vi "СПШ.vi"() -> ()   [LabVIEW 2010]
uses:
  <vilib>/Instr/_visa.llb/VISA Configure Serial Port (Instr).vi
panel:
  out "Serial Settings:Number of Bytes at Serial Port":u32
  out "x/y 2":dbl
  in  "Данные_16":i16
  in  "Данные_32":i32 format="%0.0f"
  in  "Банк":u16 format="%04x"
  out "x/y":dbl format="%#.1g"
  out "second subarray":u8[](array[numeric])
  out "Запрос":u8[](array[numeric])=[1, 5, 0, 30, 0, 0, 0, 0, 3] format="%02x"
  out "К-во байт":u16
  out "Адрес":u16=66 format="%04x"
  out "Тип":u8 format="%02x"
  in  "Тип запроса":T1(ring)
  in  "Форм.запроса":bool
  out "Смещение":i32[](array[numeric])
  out "Сорт парам":T2(array[cluster])=[{"Имя"="cp1", "Группа"="cp", "Наименование"="Пропорциональный коэффициент контура тока", "Ед. изм"=0, "Список"="", "Адрес"=0, "Описание"="Параметр настройки ПИ-регулятора контура тока", "Мин"=0, "Макс"=100, "Сервис"=TRUE, "Только чтение"=FALSE, "Разработка"=FALSE, "К-во бит"=32, "Шаг"=12, "Обработка"=FALSE, "Макрос"=""}, {"Имя"="cp2", "Группа"="cp", "Наименование"="Интегральный коэффициент контура тока", "Ед. изм"=0, "Список"="", "Адрес"=2, "Описание"="Параметр настройки ПИ-регулятора контура тока", "Мин"=0, "Макс"=200, "Сервис"=TRUE, "Только чтение"=FALSE, "Разработка"=FALSE, "К-во бит"=32, "Шаг"=12, "Обработка"=FALSE, "Макрос"=""}, {"Имя"="cp3", "Группа"="cp", "Наименование"="Максимальный ток", "Ед. изм"=1, "Список"="", "Адрес"=4, "Описание"="Определять предельную величину тока допустимую для двигателя.", "Мин"=0, "Макс"=1500, "Сервис"=FALSE, "Только чтение"=FALSE, "Разработка"=FALSE, "К-во бит"=16, "Шаг"=0, "Обработка"=TRUE, "Макрос"="macros cp3\n  ON_READ\n  READ cp3\n  cp3=cp3*5/2047\n  RETURN cp3\n  ON_WRITE\n  cp3=val*2047/5\n  WRITE cp3\nend"}, {"Имя"="cp4", "Группа"="cp", "Наименование"="Максимальная скваженность ШИМ", "Ед. изм"=1, "Список"="", "Адрес"=5, "Описание"="3070 дискрет соответствует 100% заполнения", "Мин"=0, "Макс"=6150, "Сервис"=FALSE, "Только чтение"=FALSE, "Разработка"=FALSE, "К-во бит"=16, "Шаг"=0, "Обработка"=TRUE, "Макрос"="macros cp4\n  ON_READ\n  READ cp4\n  cp4=cp4*5/2500\n  RETURN cp4\n  ON_WRITE\n  cp4=val*2500/5\n  WRITE cp4\nend"}, {"Имя"="vp1", "Группа"="vp", "Наименование"="Пропорциональный коэффициент контура скорости", "Ед. изм"=0, "Список"="", "Адрес"=6, "Описание"="Параметр настройки ПИ-регулятора контура скорости", "Мин"=0, "Макс"=60000, "Сервис"=TRUE, "Только чтение"=FALSE, "Разработка"=FALSE, "К-во бит"=32, "Шаг"=12, "Обработка"=FALSE, "Макрос"=""}, {"Имя"="vp2", "Группа"="vp", "Наименование"="Интегральный коэффициент контура скорости", "Ед. изм"=0, "Список"="", "Адрес"=7, "Описание"="Параметр настройки ПИ-регулятора контура скорости", "Мин"=0, "Макс"=60000, "Сервис"=TRUE, "Только чтение"=FALSE, "Разработка"=FALSE, "К-во бит"=32, "Шаг"=12, "Обработка"=FALSE, "Макрос"=""}, {"Имя"="vp16", "Группа"="vp", "Наименование"="Дифференциальный коэффициент контура скорости", "Ед. изм"=0, "Список"="", "Адрес"=80, "Описание"="Параметр настройки ПИ-регулятора контура скорости", "Мин"=0, "Макс"=60000, "Сервис"=TRUE, "Только чтение"=FALSE, "Разработка"=FALSE, "К-во бит"=32, "Шаг"=12, "Обработка"=FALSE, "Макрос"=""}, {"Имя"="vp3", "Группа"="vp", "Наименование"="Коэффициент обратной связи по скорости", "Ед. изм"=0, "Список"="", "Адрес"=8, "Описание"="Определяет масштаб датчика скорости", "Мин"=-1, "Макс"=1, "Сервис"=TRUE, "Только чтение"=FALSE, "Разработка"=FALSE, "К-во бит"=32, "Шаг"=12, "Обработка"=FALSE, "Макрос"=""}, {"Имя"="vp4", "Группа"="vp", "Наименование"="Частота дискретизации контура скорости", "Ед. изм"=0, "Список"="100:100\n 200:200\n 500:500\n 1000:1000\n 2000:2000\n 3000:3000\n 4000:4000\n 5000:5000\n\r\n", "Адрес"=9, "Описание"="Определяет частоту обсчета контура скорости", "Мин"=100, "Макс"=5000, "Сервис"=FALSE, "Только чтение"=FALSE, "Разработка"=FALSE, "К-во бит"=16, "Шаг"=0, "Обработка"=FALSE, "Макрос"=""}, {"Имя"="vp5", "Группа"="vp", "Наименование"="Ускорение", "Ед. изм"=2, "Список"="", "Адрес"=10, "Описание"="Определяет динамику контура скорости", "Мин"=1, "Макс"=2000000, "Сервис"=TRUE, "Только чтение"=FALSE, "Разработка"=FALSE, "К-во бит"=32, "Шаг"=10, "Обработка"=FALSE, "Макрос"=""}, {"Имя"="pp1", "Группа"="pp", "Наименование"="Пропорциональный коэффициент контура положения", "Ед. изм"=0, "Список"="", "Адрес"=11, "Описание"="Параметр настройки ПИ-регулятора контура позиционирования", "Мин"=0, "Макс"=10000, "Сервис"=TRUE, "Только чтение"=FALSE, "Разработка"=FALSE, "К-во бит"=32, "Шаг"=4, "Обработка"=FALSE, "Макрос"=""}, {"Имя"="pp2", "Группа"="pp", "Наименование"="Интегральный коэффициент контура положения", "Ед. изм"=0, "Список"="", "Адрес"=12, "Описание"="Параметр настройки ПИ-регулятора контура позиционирования", "Мин"=0, "Макс"=30000, "Сервис"=TRUE, "Только чтение"=FALSE, "Разработка"=FALSE, "К-во бит"=32, "Шаг"=4, "Обработка"=FALSE, "Макрос"=""}, {"Имя"="pp3", "Группа"="pp", "Наименование"="Частота дискретизации контура положения", "Ед. изм"=0, "Список"="25:25\n50:50\n100:100\n200:200\n500:500\n1000:1000\n2000:2000\n3000:3000\n4000:4000\n5000:5000\n\r\n", "Адрес"=13, "Описание"="Определяет частоту обсчета контура позиции.", "Мин"=25, "Макс"=5000, "Сервис"=FALSE, "Только чтение"=FALSE, "Разработка"=FALSE, "К-во бит"=16, "Шаг"=0, "Обработка"=FALSE, "Макрос"=""}, {"Имя"="vp6", "Группа"="vp", "Наименование"="Максимальное время выхода на номинальный режим", "Ед. изм"=3, "Список"="0:Не ограничено\n1:1\n2:2\n3:3\n4:4\n5:5\n6:6\n7:7\n8:8\n9:9\n10:10\n11:11\n12:12\n13:13\n14:14\n15:15\n16:16\n17:17\n18:18\n19:19\n20:20\n21:21\n22:22\n23:23\n24:24\n25:25\n26:26\n27:27\n28:28\n29:29\n30:30\r\n", "Адрес"=14, "Описание"="Время, по истечению которого привод переходит в состояние останова, если не достигнута заданная скорость", "Мин"=0, "Макс"=30, "Сервис"=FALSE, "Только чтение"=FALSE, "Разработка"=FALSE, "К-во бит"=16, "Шаг"=1, "Обработка"=TRUE, "Макрос"="macros vp6\n  ON_READ\n  READ vp6\n  if vp4=0\n  READ vp4\n  fi\n  vp6=vp6/vp4\n  RETURN vp6\n  ON_WRITE\n  if vp4=0\n  READ vp4\n  fi\n  vp6=val*vp4\n  WRITE vp6\n  ON_ERROR\n  vp6=100000000000000\n  RETURN vp6\nend"}, {"Имя"="cp5", "Группа"="cp", "Наименование"="Состояние контура тока", "Ед. изм"=0, "Список"="0:Разомкнут\n2:Замкнут\n4:Прямое управление токами в обмотках\n5:Адаптивное упрваление\n6:Прямое раздельное управление токами в обмотках\n\r\n", "Адрес"=16, "Описание"="Обеспечивает замкнутое или разомкнутое регулирование контура тока. В стандартном режиме использования контур должен быть замкнут.", "Мин"=0, "Макс"=6, "Сервис"=FALSE, "Только чтение"=FALSE, "Разработка"=FALSE, "К-во бит"=16, "Шаг"=0, "Обработка"=FALSE, "Макрос"=""}, {"Имя"="vp7", "Группа"="vp", "Наименование"="Состояние контура скорости", "Ед. изм"=0, "Список"="0:Разомкнут\n2:Замкнут\n\r\n", "Адрес"=17, "Описание"="Обеспечивает замкнутое или разомкнутое регулирование контура скорости. Контур должен быть замкнут в режиме управления скоростью привода и в режиме управления позицией.", "Мин"=0, "Макс"=2, "Сервис"=FALSE, "Только чтение"=FALSE, "Разработка"=FALSE, "К-во бит"=16, "Шаг"=0, "Обработка"=FALSE, "Макрос"=""}, {"Имя"="pp5", "Группа"="pp", "Наименование"="Состояние контура положения", "Ед. изм"=0, "Список"="0:Разомкнут\n2:Замкнут\n\r\n", "Адрес"=18, "Описание"="Обеспечивает замкнутое или разомкнутое регулирование контура позиции", "Мин"=0, "Макс"=2, "Сервис"=FALSE, "Только чтение"=FALSE, "Разработка"=FALSE, "К-во бит"=16, "Шаг"=0, "Обработка"=FALSE, "Макрос"=""}, {"Имя"="vp8", "Группа"="vp", "Наименование"="Максимальная скорость вращения", "Ед. изм"=4, "Список"="", "Адрес"=20, "Описание"="Ограничение максимальной скорости вращения привода.", "Мин"=0, "Макс"=8000, "Сервис"=TRUE, "Только чтение"=FALSE, "Разработка"=FALSE, "К-во бит"=32, "Шаг"=12, "Обработка"=FALSE, "Макрос"=""}, {"Имя"="vp9", "Группа"="vp", "Наименование"="Динамический режим", "Ед. изм"=0, "Список"="0:Режим плавного разгона/торможения\n2:Режим с максимальной динамикой\n3:Режим G декодирования\n4:S кривая\n\r\n", "Адрес"=15, "Описание"="Включает или отключает внутренний интерполятор. В режиме управления приводов от внешнего контроллера, например, от ЧПУ, привод должен находиться в режиме с максимальной динамикой. Режим G декодирования позволяет реализовать контурное управление непосредственно группой приводов без использования внешнего контроллера.", "Мин"=0, "Макс"=4, "Сервис"=FALSE, "Только чтение"=FALSE, "Разработка"=FALSE, "К-во бит"=16, "Шаг"=0, "Обработка"=FALSE, "Макрос"=""}, {"Имя"="ss1", "Группа"="ss", "Наименование"="Тестовый параметр", "Ед. изм"=0, "Список"="", "Адрес"=19, "Описание"="", "Мин"=-65535, "Макс"=65535, "Сервис"=FALSE, "Только чтение"=FALSE, "Разработка"=TRUE, "К-во бит"=16, "Шаг"=0, "Обработка"=FALSE, "Макрос"=""}, {"Имя"="ct1", "Группа"="ct", "Наименование"="Задание тока", "Ед. изм"=5, "Список"="", "Адрес"=512, "Описание"="Сигнал управления при разомкнутом контуре скорости и положения", "Мин"=-3500, "Макс"=3500, "Сервис"=FALSE, "Только чтение"=FALSE, "Разработка"=FALSE, "К-во бит"=16, "Шаг"=0, "Обработка"=TRUE, "Макрос"="macros ct1\n  ON_READ\n  READ ct1\n  ct1=ct1*5/2500\n  RETURN ct1\n  ON_WRITE\n  ct1=val*2500/5\n  WRITE ct1\nend"}, {"Имя"="ct2", "Группа"="ct", "Наименование"="Задание скорости", "Ед. изм"=4, "Список"="", "Адрес"=514, "Описание"="Сигнал управления при разомкнутом контуре положения", "Мин"=-12000, "Макс"=12000, "Сервис"=TRUE, "Только чтение"=FALSE, "Разработка"=FALSE, "К-во бит"=32, "Шаг"=12, "Обработка"=FALSE, "Макрос"=""}, {"Имя"="ct3", "Группа"="ct", "Наименование"="Задание положения", "Ед. изм"=6, "Список"="", "Адрес"=516, "Описание"="Сигнал управления при замкнутом контуре положения", "Мин"=-2147483647, "Макс"=2147483647, "Сервис"=FALSE, "Только чтение"=FALSE, "Разработка"=FALSE, "К-во бит"=32, "Шаг"=0, "Обработка"=FALSE, "Макрос"=""}, {"Имя"="dd1", "Группа"="dd", "Наименование"="Ток в обмотке 1", "Ед. изм"=5, "Список"="", "Адрес"=1024, "Описание"="Показывает ток, протекающий в обмотке двигателя", "Мин"=-5, "Макс"=5, "Сервис"=FALSE, "Только чтение"=TRUE, "Разработка"=FALSE, "К-во бит"=16, "Шаг"=0, "Обработка"=TRUE, "Макрос"="macros dd1\n  ON_READ\n  READ dd1\n  dd1=dd1*5/2047\n  RETURN dd1\n  ON_WRITE\n  dd1=val*2047/5\n  WRITE dd1\nend"}, {"Имя"="dd6", "Группа"="dd", "Наименование"="Заданный ток в обмотке 1", "Ед. изм"=5, "Список"="", "Адрес"=1034, "Описание"="", "Мин"=-2047, "Макс"=2047, "Сервис"=FALSE, "Только чтение"=FALSE, "Разработка"=FALSE, "К-во бит"=16, "Шаг"=0, "Обработка"=TRUE, "Макрос"="macros dd6\n  ON_READ\n  READ dd6\n  dd6=dd6*5/2047\n  RETURN dd6\n  ON_WRITE\n  dd6=val*2047/5\n  WRITE dd6\nend"}, {"Имя"="dd3", "Группа"="dd", "Наименование"="Ток в обмотке 2", "Ед. изм"=5, "Список"="", "Адрес"=1029, "Описание"="Индицирует ток, протекающий в обмотке двигателя", "Мин"=-5, "Макс"=5, "Сервис"=FALSE, "Только чтение"=TRUE, "Разработка"=FALSE, "К-во бит"=16, "Шаг"=0, "Обработка"=TRUE, "Макрос"="macros dd3\n  ON_READ\n  READ dd3\n  dd3=dd3*5/2047\n  RETURN dd3\n  ON_WRITE\n  dd3=val*2047/5\n  WRITE dd3\nend"}, {"Имя"="dd9", "Группа"="dd", "Наименование"="Заданный ток в обмотке 2", "Ед. изм"=5, "Список"="", "Адрес"=1037, "Описание"="", "Мин"=-2047, "Макс"=2047, "Сервис"=FALSE, "Только чтение"=FALSE, "Разработка"=FALSE, "К-во бит"=16, "Шаг"=0, "Обработка"=TRUE, "Макрос"="macros dd9\n  ON_READ\n  READ dd9\n  dd9=dd9*5/2047\n  RETURN dd9\n  ON_WRITE\n  dd9=val*2047/5\n  WRITE dd9\nend"}, {"Имя"="dd2", "Группа"="dd", "Наименование"="Заданный ток в роторной системе координат", "Ед. изм"=5, "Список"="", "Адрес"=1026, "Описание"="Индицирует ток, который задан контуром скорости", "Мин"=-5, "Макс"=5, "Сервис"=FALSE, "Только чтение"=TRUE, "Разработка"=FALSE, "К-во бит"=16, "Шаг"=0, "Обработка"=TRUE, "Макрос"="macros dd2\n  ON_READ\n  READ dd2\n  dd2=dd2*5/2047\n  RETURN dd2\n  ON_WRITE\n  dd2=val*2047/5\n  WRITE dd2\nend"}, {"Имя"="dd4", "Группа"="dd", "Наименование"="Текущая скорость вращения", "Ед. изм"=4, "Список"="", "Адрес"=1032, "Описание"="", "Мин"=-5000, "Макс"=5000, "Сервис"=FALSE, "Только чтение"=TRUE, "Разработка"=FALSE, "К-во бит"=8, "Шаг"=12, "Обработка"=FALSE, "Макрос"=""}, {"Имя"="dd5", "Группа"="dd", "Наименование"="Заданная скорость вращения", "Ед. изм"=4, "Список"="", "Адрес"=1033, "Описание"="", "Мин"=-5000, "Макс"=5000, "Сервис"=FALSE, "Только чтение"=TRUE, "Разработка"=FALSE, "К-во бит"=16, "Шаг"=12, "Обработка"=FALSE, "Макрос"=""}, {"Имя"="dd21", "Группа"="dd", "Наименование"="Ошибка контура скорости", "Ед. изм"=4, "Список"="", "Адрес"=1049, "Описание"="", "Мин"=-65535, "Макс"=65535, "Сервис"=FALSE, "Только чтение"=TRUE, "Разработка"=FALSE, "К-во бит"=16, "Шаг"=1, "Обработка"=FALSE, "Макрос"=""}, {"Имя"="dd7", "Группа"="dd", "Наименование"="Заданная позиция", "Ед. изм"=6, "Список"="", "Адрес"=1035, "Описание"="", "Мин"=-2147483647, "Макс"=2147483647, "Сервис"=FALSE, "Только чтение"=TRUE, "Разработка"=FALSE, "К-во бит"=32, "Шаг"=0, "Обработка"=FALSE, "Макрос"=""}, {"Имя"="dd8", "Группа"="dd", "Наименование"="Текущая позиция", "Ед. изм"=6, "Список"="", "Адрес"=1036, "Описание"="", "Мин"=-2147483647, "Макс"=2147483647, "Сервис"=FALSE, "Только чтение"=TRUE, "Разработка"=FALSE, "К-во бит"=32, "Шаг"=0, "Обработка"=FALSE, "Макрос"=""}, {"Имя"="dd20", "Группа"="dd", "Наименование"="Ошибка контура позиции", "Ед. изм"=6, "Список"="", "Адрес"=1048, "Описание"="", "Мин"=-2147483647, "Макс"=2147483647, "Сервис"=TRUE, "Только чтение"=TRUE, "Разработка"=FALSE, "К-во бит"=32, "Шаг"=10, "Обработка"=FALSE, "Макрос"=""}, {"Имя"="dd10", "Группа"="dd", "Наименование"="Температура внутри корпуса", "Ед. изм"=7, "Список"="", "Адрес"=1038, "Описание"="", "Мин"=-40, "Макс"=120, "Сервис"=FALSE, "Только чтение"=TRUE, "Разработка"=FALSE, "К-во бит"=16, "Шаг"=0, "Обработка"=TRUE, "Макрос"="macros dd10\n  ON_READ\n  READ dd10\n  dd10=dd10/128\n  RETURN dd10\n  ON_WRITE\n  dd10=val\n  WRITE dd10\nend"}, {"Имя"="dd19", "Группа"="dd", "Наименование"="Текущее цифровое напряжение", "Ед. изм"=8, "Список"="", "Адрес"=1047, "Описание"="", "Мин"=0, "Макс"=23, "Сервис"=FALSE, "Только чтение"=TRUE, "Разработка"=FALSE, "К-во бит"=16, "Шаг"=0, "Обработка"=TRUE, "Макрос"="macros dd19\n  ON_READ\n  READ dd19\n  dd19=dd19/178\n  RETURN dd19\n  ON_WRITE\n  dd19=val\n  WRITE dd19\nend"}, {"Имя"="dd12", "Группа"="dd", "Наименование"="Текущее напряжение питания", "Ед. изм"=8, "Список"="", "Адрес"=1040, "Описание"="", "Мин"=0, "Макс"=120, "Сервис"=FALSE, "Только чтение"=TRUE, "Разработка"=FALSE, "К-во бит"=16, "Шаг"=0, "Обработка"=TRUE, "Макрос"="macros dd12\n  ON_READ\n  READ dd12\n  dd12=dd12/21\n  RETURN dd12\n  ON_WRITE\n  dd12=val\n  WRITE dd12\nend"}, {"Имя"="dd11", "Группа"="dd", "Наименование"="Статус контроллера", "Ед. изм"=0, "Список"="0:Исправен\n1:Останов по команде\n2:Останов - высокое противодействующее усилие\n3:Останов - короткое замыкание\n4:Выход из температурного диапазона\n5:Повышенное силовое напряжение\n6:Низкое силовое напряжение\n7:Повышенное цифровое напряжение\n8:Низкое цифровое напряжение\n9:Cиловое напряжение превышает напряжение, установл. пользователем\n10:Останов - превышение допустимой перегрузки\n11:Останов - сработала защита IGBT модуля\n12:Останов - Ошибка поиска фазы по UVW трекам\n13:Останов - ошибка в настройках энкодера\n14: Останов - сбой в работе энкодера\n15: Останов - Ошибка фазировки двигателя\n\r\n", "Адрес"=1039, "Описание"="Привод в состоянии отработать задание только, если его статус \"Исправен\".", "Мин"=0, "Макс"=15, "Сервис"=FALSE, "Только чтение"=FALSE, "Разработка"=FALSE, "К-во бит"=16, "Шаг"=0, "Обработка"=FALSE, "Макрос"=""}, {"Имя"="st1", "Группа"="st", "Наименование"="Разрешение", "Ед. изм"=6, "Список"="", "Адрес"=21, "Описание"="Разрешение датчика положения/скорости", "Мин"=0, "Макс"=2147483647, "Сервис"=FALSE, "Только чтение"=FALSE, "Разработка"=FALSE, "К-во бит"=32, "Шаг"=0, "Обработка"=FALSE, "Макрос"=""}, {"Имя"="tp1", "Группа"="tp", "Наименование"="Режим осциллографа", "Ед. изм"=0, "Список"="0:Непрерывный режим\n1:Ступенька\n2:Синус\n3:Приращение скорости\n4:Синусоидальное изменение скорости\n5:Треугольное изменение позиции\n6:Измерение без задания\n7:Измерение без задания до принудительного останова\n8:Приращение момента\n\r\n", "Адрес"=1280, "Описание"="Режим сканирования динамических параметров (отображение выбранных параметров в процессе работы привода).", "Мин"=0, "Макс"=8, "Сервис"=FALSE, "Только чтение"=FALSE, "Разработка"=FALSE, "К-во бит"=16, "Шаг"=0, "Обработка"=FALSE, "Макрос"=""}, {"Имя"="tp3", "Группа"="tp", "Наименование"="Амплитуда задания положения", "Ед. изм"=0, "Список"="", "Адрес"=1284, "Описание"="Определяет величину приращения позиции в режиме осциллографа 1.", "Мин"=-2147483647, "Макс"=2147483647, "Сервис"=FALSE, "Только чтение"=FALSE, "Разработка"=FALSE, "К-во бит"=32, "Шаг"=0, "Обработка"=FALSE, "Макрос"=""}, {"Имя"="ip0", "Группа"="ip", "Наименование"="Источник опорного сигнала", "Ед. изм"=0, "Список"="0:Интерфейс USB\n2:Интерфейс StepDir\n4:Аналоговый интерфейс\n5:Интерфейс CAN\n6:Квадратурный интерфейс\r\n", "Адрес"=23, "Описание"="Определяет интерфейс, по которому осуществляется ввод задания для привода.", "Мин"=0, "Макс"=6, "Сервис"=FALSE, "Только чтение"=FALSE, "Разработка"=FALSE, "К-во бит"=16, "Шаг"=0, "Обработка"=FALSE, "Макрос"=""}, {"Имя"="st2", "Группа"="st", "Наименование"="Версия ПО драйвера", "Ед. изм"=0, "Список"="", "Адрес"=22, "Описание"="Текущая версия программного обеспечения привода.", "Мин"=0, "Макс"=2147483647, "Сервис"=TRUE, "Только чтение"=FALSE, "Разработка"=FALSE, "К-во бит"=32, "Шаг"=12, "Обработка"=FALSE, "Макрос"=""}, {"Имя"="ip1", "Группа"="ip", "Наименование"="Коэффициент веса одной дискреты", "Ед. изм"=0, "Список"="", "Адрес"=24, "Описание"="Определяет количество импульсов датчика, на которые необходимо повернуть вал двигателя, при получении одной дискреты по интерфейсу Step/Dir, т.е. масштаб одного импульса", "Мин"=-4000, "Макс"=4000, "Сервис"=TRUE, "Только чтение"=FALSE, "Разработка"=FALSE, "К-во бит"=32, "Шаг"=10, "Обработка"=FALSE, "Макрос"=""}, {"Имя"="tp2", "Группа"="tp", "Наименование"="Период опроса параметров", "Ед. изм"=9, "Список"="", "Адрес"=1282, "Описание"="Определяет интервал времени между запоминанием данных в массив в режимах 1-7.", "Мин"=25, "Макс"=25000, "Сервис"=FALSE, "Только чтение"=FALSE, "Разработка"=FALSE, "К-во бит"=16, "Шаг"=25, "Обработка"=FALSE, "Макрос"=""}, {"Имя"="tp5", "Группа"="tp", "Наименование"="Период задающего воздействия", "Ед. изм"=9, "Список"="", "Адрес"=1285, "Описание"="Данный параметр определяет задержку введения задающего воздействия от начала сбора информации в режиме осциллографа 1 и 3.", "Мин"=25, "Макс"=800000, "Сервис"=FALSE, "Только чтение"=FALSE, "Разработка"=FALSE, "К-во бит"=16, "Шаг"=25, "Обработка"=TRUE, "Макрос"="macros tp5\n  ON_READ\n  READ tp5\n  tp5=tp5*25\n  RETURN tp5\n  ON_WRITE\n  tp5=val/25\n  WRITE tp5\n  ON_ERROR\n  err=100000000000\n  RETURN err\nend"}, {"Имя"="tp6", "Группа"="tp", "Наименование"="Амплитуда задания скорости", "Ед. изм"=4, "Список"="", "Адрес"=1286, "Описание"="Определяет величину приращения скорости в режиме осциллографа 3.", "Мин"=-14000, "Макс"=14000, "Сервис"=FALSE, "Только чтение"=FALSE, "Разработка"=FALSE, "К-во бит"=16, "Шаг"=0, "Обработка"=FALSE, "Макрос"=""}, {"Имя"="ip2", "Группа"="ip", "Наименование"="Текущий банк программы интерпретатора", "Ед. изм"=10, "Список"="0:0\n1:1\n2:2\n3:3\n4:4\n5:5\n6:6\n7:7\n255:Программа не выбрана\n\r\n", "Адрес"=26, "Описание"="Банк, из которой загружена программа на выполнение.", "Мин"=0, "Макс"=255, "Сервис"=FALSE, "Только чтение"=FALSE, "Разработка"=FALSE, "К-во бит"=16, "Шаг"=1, "Обработка"=FALSE, "Макрос"=""}, {"Имя"="ip3", "Группа"="ip", "Наименование"="Текущий банк чт/записи программ интерпретатора", "Ед. изм"=10, "Список"="0:0\n1:1\n2:2\n3:3\n4:4\n5:5\n6:6\n7:7\n255:Программа не выбрана\n\r\n", "Адрес"=27, "Описание"="", "Мин"=0, "Макс"=255, "Сервис"=FALSE, "Только чтение"=TRUE, "Разработка"=TRUE, "К-во бит"=16, "Шаг"=1, "Обработка"=FALSE, "Макрос"=""}, {"Имя"="ip4", "Группа"="ip", "Наименование"="Режим работы интерпретатора", "Ед. изм"=0, "Список"="0:Режим выполнения программы\n1:Режим отладки\n\r\n", "Адрес"=28, "Описание"="Режим работы интерпретатора", "Мин"=0, "Макс"=1, "Сервис"=FALSE, "Только чтение"=FALSE, "Разработка"=FALSE, "К-во бит"=16, "Шаг"=1, "Обработка"=FALSE, "Макрос"=""}, {"Имя"="st3", "Группа"="st", "Наименование"="Уникальный идентификатор устройства", "Ед. изм"=0, "Список"="", "Адрес"=30, "Описание"="", "Мин"=0, "Макс"=2147483647, "Сервис"=FALSE, "Только чтение"=FALSE, "Разработка"=FALSE, "К-во бит"=32, "Шаг"=0, "Обработка"=FALSE, "Макрос"=""}, {"Имя"="ip5", "Группа"="ip", "Наименование"="Порт ввода вывода", "Ед. изм"=0, "Список"="", "Адрес"=29, "Описание"="Старший байт содержит содержимое порта вывода, младший - состояние линий ввода.", "Мин"=0, "Макс"=65535, "Сервис"=FALSE, "Только чтение"=FALSE, "Разработка"=FALSE, "К-во бит"=16, "Шаг"=0, "Обработка"=FALSE, "Макрос"=""}, {"Имя"="ss2", "Группа"="ss", "Наименование"="Количество КЗ", "Ед. изм"=0, "Список"="", "Адрес"=31, "Описание"="Количество зафиксированных коротких замыканий", "Мин"=0, "Макс"=65535, "Сервис"=FALSE, "Только чтение"=FALSE, "Разработка"=FALSE, "К-во бит"=16, "Шаг"=0, "Обработка"=FALSE, "Макрос"=""}, {"Имя"="ss3", "Группа"="ss", "Наименование"="Количество превышений температуры", "Ед. изм"=0, "Список"="", "Адрес"=32, "Описание"="Количество зафиксированных превышений температуры", "Мин"=0, "Макс"=65535, "Сервис"=FALSE, "Только чтение"=FALSE, "Разработка"=FALSE, "К-во бит"=16, "Шаг"=0, "Обработка"=FALSE, "Макрос"=""}, {"Имя"="ss4", "Группа"="ss", "Наименование"="Количество перенапряжений", "Ед. изм"=0, "Список"="", "Адрес"=33, "Описание"="Количество зафиксированных перенапряжений", "Мин"=0, "Макс"=65535, "Сервис"=FALSE, "Только чтение"=FALSE, "Разработка"=FALSE, "К-во бит"=16, "Шаг"=0, "Обработка"=FALSE, "Макрос"=""}, {"Имя"="ss5", "Группа"="ss", "Наименование"="Количество недонапряжений", "Ед. изм"=0, "Список"="", "Адрес"=34, "Описание"="Количество зафиксированных случаев пониженного напряжений", "Мин"=0, "Макс"=65535, "Сервис"=FALSE, "Только чтение"=FALSE, "Разработка"=FALSE, "К-во бит"=16, "Шаг"=0, "Обработка"=FALSE, "Макрос"=""}, {"Имя"="ss6", "Группа"="ss", "Наименование"="Количество перегрузок", "Ед. изм"=0, "Список"="", "Адрес"=35, "Описание"="", "Мин"=0, "Макс"=65535, "Сервис"=FALSE, "Только чтение"=FALSE, "Разработка"=FALSE, "К-во бит"=16, "Шаг"=0, "Обработка"=FALSE, "Макрос"=""}, {"Имя"="ss7", "Группа"="ss", "Наименование"="Количество перепрогарммирований", "Ед. изм"=0, "Список"="", "Адрес"=36, "Описание"="", "Мин"=0, "Макс"=65535, "Сервис"=FALSE, "Только чтение"=FALSE, "Разработка"=FALSE, "К-во бит"=16, "Шаг"=0, "Обработка"=FALSE, "Макрос"=""}, {"Имя"="ss8", "Группа"="ss", "Наименование"="Сообщение 0", "Ед. изм"=0, "Список"="1:Короткое замыкание\n2:Перегрев\n3:Повышенное напряжение\n4:Пониженное напряжение\n5:Перегрузка по току\n6:Произведена перезапись контроллера\n\r\n", "Адрес"=37, "Описание"="Журнал последних 8 сообщений", "Мин"=0, "Макс"=65535, "Сервис"=FALSE, "Только чтение"=FALSE, "Разработка"=FALSE, "К-во бит"=16, "Шаг"=0, "Обработка"=FALSE, "Макрос"=""}, {"Имя"="ss9", "Группа"="ss", "Наименование"="Сообщение 1", "Ед. изм"=0, "Список"="1:Короткое замыкание\n2:Перегрев\n3:Повышенное напряжение\n4:Пониженное напряжение\n5:Перегрузка по току\n6:Произведена перезапись контроллера\n\r\n", "Адрес"=38, "Описание"="Журнал последних 8 сообщений", "Мин"=0, "Макс"=65535, "Сервис"=FALSE, "Только чтение"=FALSE, "Разработка"=FALSE, "К-во бит"=16, "Шаг"=0, "Обработка"=FALSE, "Макрос"=""}, {"Имя"="ss10", "Группа"="ss", "Наименование"="Сообщение 2", "Ед. изм"=0, "Список"="1:Короткое замыкание\n2:Перегрев\n3:Повышенное напряжение\n4:Пониженное напряжение\n5:Перегрузка по току\n6:Произведена перезапись контроллера\n\r\n", "Адрес"=39, "Описание"="Журнал последних 8 сообщений", "Мин"=0, "Макс"=65535, "Сервис"=FALSE, "Только чтение"=FALSE, "Разработка"=FALSE, "К-во бит"=16, "Шаг"=0, "Обработка"=FALSE, "Макрос"=""}, {"Имя"="ss11", "Группа"="ss", "Наименование"="Сообщение 3", "Ед. изм"=0, "Список"="1:Короткое замыкание\n2:Перегрев\n3:Повышенное напряжение\n4:Пониженное напряжение\n5:Перегрузка по току\n6:Произведена перезапись контроллера\n\r\n", "Адрес"=40, "Описание"="Журнал последних 8 сообщений", "Мин"=0, "Макс"=65535, "Сервис"=FALSE, "Только чтение"=FALSE, "Разработка"=FALSE, "К-во бит"=16, "Шаг"=0, "Обработка"=FALSE, "Макрос"=""}, {"Имя"="ss12", "Группа"="ss", "Наименование"="Сообщение 4", "Ед. изм"=0, "Список"="1:Короткое замыкание\n2:Перегрев\n3:Повышенное напряжение\n4:Пониженное напряжение\n5:Перегрузка по току\n6:Произведена перезапись контроллера\n\r\n", "Адрес"=41, "Описание"="Журнал последних 8 сообщений", "Мин"=0, "Макс"=65535, "Сервис"=FALSE, "Только чтение"=FALSE, "Разработка"=FALSE, "К-во бит"=16, "Шаг"=0, "Обработка"=FALSE, "Макрос"=""}, {"Имя"="ss13", "Группа"="ss", "Наименование"="Сообщение 5", "Ед. изм"=0, "Список"="1:Короткое замыкание\n2:Перегрев\n3:Повышенное напряжение\n4:Пониженное напряжение\n5:Перегрузка по току\n6:Произведена перезапись контроллера\n\r\n", "Адрес"=42, "Описание"="Журнал последних 8 сообщений", "Мин"=0, "Макс"=65535, "Сервис"=FALSE, "Только чтение"=FALSE, "Разработка"=FALSE, "К-во бит"=16, "Шаг"=0, "Обработка"=FALSE, "Макрос"=""}, {"Имя"="ss14", "Группа"="ss", "Наименование"="Сообщение 6", "Ед. изм"=0, "Список"="1:Короткое замыкание\n2:Перегрев\n3:Повышенное напряжение\n4:Пониженное напряжение\n5:Перегрузка по току\n6:Произведена перезапись контроллера\n\r\n", "Адрес"=43, "Описание"="Журнал последних 8 сообщений", "Мин"=0, "Макс"=65535, "Сервис"=FALSE, "Только чтение"=FALSE, "Разработка"=FALSE, "К-во бит"=16, "Шаг"=0, "Обработка"=FALSE, "Макрос"=""}, {"Имя"="ss15", "Группа"="ss", "Наименование"="Сообщение 7", "Ед. изм"=0, "Список"="1:Короткое замыкание\n2:Перегрев\n3:Повышенное напряжение\n4:Пониженное напряжение\n5:Перегрузка по току\n6:Произведена перезапись контроллера\n\r\n", "Адрес"=44, "Описание"="Журнал последних 8 сообщений", "Мин"=0, "Макс"=65535, "Сервис"=FALSE, "Только чтение"=FALSE, "Разработка"=FALSE, "К-во бит"=16, "Шаг"=0, "Обработка"=FALSE, "Макрос"=""}, {"Имя"="ip6", "Группа"="ip", "Наименование"="Смещение диапазона сигнала управления", "Ед. изм"=0, "Список"="", "Адрес"=48, "Описание"="Используется для корректировки диапазона регулирования входного сигнала (аналогового или Step\\Dir). Значение 2048 соответствует нулевой скорости при подаче на вход нулевого напряжения.", "Мин"=0, "Макс"=4096, "Сервис"=FALSE, "Только чтение"=FALSE, "Разработка"=FALSE, "К-во бит"=16, "Шаг"=0, "Обработка"=FALSE, "Макрос"=""}, {"Имя"="dd13", "Группа"="dd", "Наименование"="Тестовый параметр 1", "Ед. изм"=0, "Список"="", "Адрес"=1041, "Описание"="Пока используется для индикации перехода на меандр вместо синуса. Параметр для разработчика", "Мин"=-65535, "Макс"=65535, "Сервис"=FALSE, "Только чтение"=TRUE, "Разработка"=TRUE, "К-во бит"=16, "Шаг"=0, "Обработка"=FALSE, "Макрос"=""}, {"Имя"="dd14", "Группа"="dd", "Наименование"="Тестовый параметр 2", "Ед. изм"=0, "Список"="", "Адрес"=1042, "Описание"="Пока используется для индикации сдвига фазы", "Мин"=-65535, "Макс"=65535, "Сервис"=FALSE, "Только чтение"=TRUE, "Разработка"=TRUE, "К-во бит"=16, "Шаг"=0, "Обработка"=FALSE, "Макрос"=""}, {"Имя"="vp10", "Группа"="vp", "Наименование"="Начало резонансного диапазона 1", "Ед. изм"=4, "Список"="", "Адрес"=49, "Описание"="Если начало и конец диапазона равны, то диапазон не выбран.", "Мин"=0, "Макс"=8000, "Сервис"=FALSE, "Только чтение"=FALSE, "Разработка"=FALSE, "К-во бит"=16, "Шаг"=0, "Обработка"=TRUE, "Макрос"="macros vp10\n  ON_READ\n  READ vp10\n  if st1=0\n  READ st1\n  fi\n  if vp4=0\n  READ vp4\n  fi\n  if vp3=0\n  READ vp3\n  fi\n  vp10=round(60*vp10*vp4/(st1*vp3))\n  RETURN vp10\n  ON_WRITE\n  if st1=0\n  READ st1\n  fi\n  if vp4=0\n  READ vp4\n  fi\n  if vp3=0\n  READ vp3\n  fi\n  vp10=val*st1*vp3/(60*vp4)\n  WRITE vp10\n  ON_ERROR\n  vp10=100000000000000\n  RETURN vp10\nend"}, {"Имя"="vp11", "Группа"="vp", "Наименование"="Конец резонансного диапазона 1", "Ед. изм"=4, "Список"="", "Адрес"=50, "Описание"="Если начало и конец диапазона равны, то диапазон не выбран.", "Мин"=0, "Макс"=8000, "Сервис"=FALSE, "Только чтение"=FALSE, "Разработка"=FALSE, "К-во бит"=16, "Шаг"=0, "Обработка"=TRUE, "Макрос"="macros vp11\n  ON_READ\n  READ vp11\n  if st1=0\n  READ st1\n  fi\n  if vp4=0\n  READ vp4\n  fi\n  if vp3=0\n  READ vp3\n  fi\n  vp11=round(60*vp11*vp4/(st1*vp3))\n  RETURN vp11\n  ON_WRITE\n  if st1=0\n  READ st1\n  fi\n  if vp4=0\n  READ vp4\n  fi\n  if vp3=0\n  READ vp3\n  fi\n  vp11=val*st1*vp3/(60*vp4)\n  WRITE vp11\n  ON_ERROR\n  vp11=100000000000000\n  RETURN vp11\nend"}, {"Имя"="vp12", "Группа"="vp", "Наименование"="Начало резонансного диапазона 2", "Ед. изм"=4, "Список"="", "Адрес"=51, "Описание"="Если начало и конец диапазона равны, то диапазон не выбран.", "Мин"=0, "Макс"=8000, "Сервис"=FALSE, "Только чтение"=FALSE, "Разработка"=FALSE, "К-во бит"=16, "Шаг"=0, "Обработка"=TRUE, "Макрос"="macros vp12\n  ON_READ\n  READ vp12\n  if st1=0\n  READ st1\n  fi\n  if vp4=0\n  READ vp4\n  fi\n  if vp3=0\n  READ vp3\n  fi\n  vp12=round(60*vp12*vp4/(st1*vp3))\n  RETURN vp12\n  ON_WRITE\n  if st1=0\n  READ st1\n  fi\n  if vp4=0\n  READ vp4\n  fi\n  if vp3=0\n  READ vp3\n  fi\n  vp12=val*st1*vp3/(60*vp4)\n  WRITE vp12\n  ON_ERROR\n  vp12=100000000000000\n  RETURN vp12\nend"}, {"Имя"="vp13", "Группа"="vp", "Наименование"="Конец резонансного диапазона 2", "Ед. изм"=4, "Список"="", "Адрес"=52, "Описание"="Если начало и конец диапазона равны, то диапазон не выбран.", "Мин"=0, "Макс"=8000, "Сервис"=FALSE, "Только чтение"=FALSE, "Разработка"=FALSE, "К-во бит"=16, "Шаг"=0, "Обработка"=TRUE, "Макрос"="macros vp13\n  ON_READ\n  READ vp13\n  if st1=0\n  READ st1\n  fi\n  if vp4=0\n  READ vp4\n  fi\n  if vp3=0\n  READ vp3\n  fi\n  vp13=round(60*vp13*vp4/(st1*vp3))\n  RETURN vp13\n  ON_WRITE\n  if st1=0\n  READ st1\n  fi\n  if vp4=0\n  READ vp4\n  fi\n  if vp3=0\n  READ vp3\n  fi\n  vp13=val*st1*vp3/(60*vp4)\n  WRITE vp13\n  ON_ERROR\n  vp13=100000000000000\n  RETURN vp13\nend"}, {"Имя"="ip7", "Группа"="ip", "Наименование"="CAN адрес устройства", "Ед. изм"=0, "Список"="", "Адрес"=53, "Описание"="Адрес данного устройства в сети CAN", "Мин"=0, "Макс"=127, "Сервис"=FALSE, "Только чтение"=FALSE, "Разработка"=FALSE, "К-во бит"=16, "Шаг"=0, "Обработка"=FALSE, "Макрос"=""}, {"Имя"="ip8", "Группа"="ip", "Наименование"="CAN адрес удаленного узла", "Ед. изм"=0, "Список"="", "Адрес"=54, "Описание"="Адрес удаленного устройства в сети CAN, которое выступает в качестве мастера для данного устройства", "Мин"=0, "Макс"=127, "Сервис"=FALSE, "Только чтение"=FALSE, "Разработка"=FALSE, "К-во бит"=16, "Шаг"=0, "Обработка"=FALSE, "Макрос"=""}, {"Имя"="ip9", "Группа"="ip", "Наименование"="Режим синхронизации по CAN", "Ед. изм"=0, "Список"="0:Режим не выбран\n1:Режим мастер\n2:Режим слейв\n3:Режим контурного управления\n4:Синхронизация по команде SYNC\n\r\n", "Адрес"=55, "Описание"="В режиме мастер привод передает текущую позицию в CAN на адрес удаленного узла.", "Мин"=0, "Макс"=4, "Сервис"=FALSE, "Только чтение"=FALSE, "Разработка"=FALSE, "К-во бит"=16, "Шаг"=0, "Обработка"=FALSE, "Макрос"=""}, {"Имя"="ip10", "Группа"="ip", "Наименование"="Статус шины CAN", "Ед. изм"=0, "Список"="0:Норма\n1:Неисправности на линии\n2:Ошибка передачи синхронизации слейву\n3:Ошибка - подтверждение не получено.\r\n", "Адрес"=56, "Описание"="Статус 2 - устанавливается, если мастер не может передать сообщение слейву в течение ip7", "Мин"=0, "Макс"=3, "Сервис"=FALSE, "Только чтение"=TRUE, "Разработка"=FALSE, "К-во бит"=16, "Шаг"=0, "Обработка"=FALSE, "Макрос"=""}, {"Имя"="vp14", "Группа"="vp", "Наименование"="Номинальная скорость", "Ед. изм"=4, "Список"="", "Адрес"=57, "Описание"="Скорость, начиная с которой выполняется режим ослабления поля.", "Мин"=0, "Макс"=5000, "Сервис"=FALSE, "Только чтение"=FALSE, "Разработка"=FALSE, "К-во бит"=16, "Шаг"=0, "Обработка"=TRUE, "Макрос"="macros vp14\n  ON_READ\n  READ vp14\n  if st1=0\n  READ st1\n  fi\n  if vp4=0\n  READ vp4\n  fi\n  x=round(60*vp14*1000/4000)\n  RETURN x\n  ON_WRITE\n  if st1=0\n  READ st1\n  fi\n  if vp4=0\n  READ vp4\n  fi\n  vp14=val*4000/(60*1000)\n  WRITE vp14\n  ON_STREAM_REQ\n  READ st1\n  READ vp4\n  ON_ERROR\n  dd4=100000000000000\n  RETURN vp14\nend"}, {"Имя"="vp15", "Группа"="vp", "Наименование"="Авто расчет номинальной скорости", "Ед. изм"=0, "Список"="1:Да\n0:Нет\n\r\n", "Адрес"=64, "Описание"="Автоматический расчет номинальной скорости выполняется на основе текущего напряжения питания при включении привода.", "Мин"=0, "Макс"=1, "Сервис"=FALSE, "Только чтение"=FALSE, "Разработка"=FALSE, "К-во бит"=16, "Шаг"=0, "Обработка"=FALSE, "Макрос"=""}, {"Имя"="si1", "Группа"="ss", "Наименование"="Смещение датчика тока 1", "Ед. изм"=0, "Список"="", "Адрес"=1536, "Описание"="Формула расчета I=cur1-511-si1", "Мин"=0, "Макс"=4096, "Сервис"=FALSE, "Только чтение"=FALSE, "Разработка"=TRUE, "К-во бит"=16, "Шаг"=0, "Обработка"=FALSE, "Макрос"=""}, {"Имя"="si2", "Группа"="ss", "Наименование"="Смещение датчика тока 2", "Ед. изм"=0, "Список"="", "Адрес"=1537, "Описание"="Формула расчета I=cur2-511-si2", "Мин"=0, "Макс"=4096, "Сервис"=FALSE, "Только чтение"=FALSE, "Разработка"=TRUE, "К-во бит"=16, "Шаг"=0, "Обработка"=FALSE, "Макрос"=""}, {"Имя"="pp6", "Группа"="pp", "Наименование"="Ограничение интегральной составляющей контура позиции", "Ед. изм"=0, "Список"="", "Адрес"=65, "Описание"="Определяет максимальное значение, до которого может увеличиваться интегральная составляющая. По достижению этой величины интегральная составляющая удерживается константой.", "Мин"=0, "Макс"=15000, "Сервис"=TRUE, "Только чтение"=FALSE, "Разработка"=FALSE, "К-во бит"=32, "Шаг"=10, "Обработка"=FALSE, "Макрос"=""}, {"Имя"="ip11", "Группа"="ip", "Наименование"="Статус интерпретатора", "Ед. изм"=0, "Список"="0:Норма\n1:Смена банка программ\n2:Неизвестный параметр\n3:Неизвестная команда\n4:Останов\n5:STATUS_UNKNOWN_AL_OP\n6:STATUS_UNKNOWN_CMP_OP\n7:Загрузка программы\n8:STATUS_DEBUG_BREAK\n9:STATUS_DEBUG_WAIT_END_OF_CMD\n10:Неизвестная динамическая функция\n11:Старая версия программы\n12:Слишком много циклов\n77:Неправильное условие\n13:Не удалось найти Z метку\n78:Переполнение стека\n79:Попытка чтения пустого стека\n\r\n", "Адрес"=66, "Описание"="", "Мин"=0, "Макс"=12, "Сервис"=FALSE, "Только чтение"=TRUE, "Разработка"=FALSE, "К-во бит"=16, "Шаг"=1, "Обработка"=FALSE, "Макрос"=""}, {"Имя"="ep1", "Группа"="ep", "Наименование"="Режим торможения", "Ед. изм"=0, "Список"="0:Торможение без контроля напряжения\n2:Торможение с контролем напряжения\n\r\n", "Адрес"=67, "Описание"="При торможении без контроля напряжения привод перейдет в аварийное состояние в момент превышения напряжением допустимого значения, установленным в параметре ep2.", "Мин"=0, "Макс"=2, "Сервис"=FALSE, "Только чтение"=FALSE, "Разработка"=FALSE, "К-во бит"=16, "Шаг"=0, "Обработка"=FALSE, "Макрос"=""}, {"Имя"="ep2", "Группа"="ep", "Наименование"="Максимальное напряжение", "Ед. изм"=8, "Список"="", "Адрес"=68, "Описание"="Максимальное допустимое напряжение, при котором привод должен переходить в состояние отключения.", "Мин"=0, "Макс"=280, "Сервис"=FALSE, "Только чтение"=FALSE, "Разработка"=FALSE, "К-во бит"=16, "Шаг"=0, "Обработка"=TRUE, "Макрос"="macros ep2\n  ON_READ\n  READ ep2\n  ep2=ep2/21\n  RETURN ep2\n  ON_WRITE\n  ep2=val*21\n  WRITE ep2\nend"}, {"Имя"="dd15", "Группа"="dd", "Наименование"="Время выполнения команды интерпретатором", "Ед. изм"=11, "Список"="", "Адрес"=1043, "Описание"="Определяет максимальное время, которое интерпретатор затрачивает на выполнение команды в текущей программе.", "Мин"=0, "Макс"=2147483647, "Сервис"=FALSE, "Только чтение"=TRUE, "Разработка"=FALSE, "К-во бит"=32, "Шаг"=1, "Обработка"=TRUE, "Макрос"="macros dd15\n  ON_READ\n  READ dd15\n  dd15=dd15*25/1000\n  RETURN dd15\n  ON_WRITE\n  dd15=val\n  WRITE dd15\nend"}, {"Имя"="dd16", "Группа"="dd", "Наименование"="Время выполнения программы интерпретатором", "Ед. изм"=11, "Список"="", "Адрес"=1044, "Описание"="Определяет максимальное время, которое интерпретатор затрачивает на выполнение всей программы.", "Мин"=0, "Макс"=2147483647, "Сервис"=FALSE, "Только чтение"=TRUE, "Разработка"=FALSE, "К-во бит"=32, "Шаг"=1, "Обработка"=TRUE, "Макрос"="macros dd16\n  ON_READ\n  READ dd16\n  dd16=dd16*25/1000\n  RETURN dd16\n  ON_WRITE\n  dd16=val\n  WRITE dd16\nend"}, {"Имя"="ip12", "Группа"="ip", "Наименование"="Мертвая зона аналоговых входов", "Ед. изм"=1, "Список"="", "Адрес"=69, "Описание"="Определяет зону нечувствительности аналоговых входов привода. При ручном управлении, например, с помощью джойстика, данный параметр позволяет исключить вращение вала при задании нулевой скорости.", "Мин"=0, "Макс"=250, "Сервис"=FALSE, "Только чтение"=FALSE, "Разработка"=FALSE, "К-во бит"=16, "Шаг"=0, "Обработка"=FALSE, "Макрос"=""}, {"Имя"="dd17", "Группа"="dd", "Наименование"="Аналоговый вход 0", "Ед. изм"=1, "Список"="", "Адрес"=1045, "Описание"="", "Мин"=-65535, "Макс"=65535, "Сервис"=FALSE, "Только чтение"=TRUE, "Разработка"=FALSE, "К-во бит"=16, "Шаг"=0, "Обработка"=FALSE, "Макрос"=""}, {"Имя"="dd18", "Группа"="dd", "Наименование"="Аналоговый вход 1", "Ед. изм"=1, "Список"="", "Адрес"=1046, "Описание"="", "Мин"=-65535, "Макс"=65535, "Сервис"=FALSE, "Только чтение"=TRUE, "Разработка"=FALSE, "К-во бит"=16, "Шаг"=0, "Обработка"=FALSE, "Макрос"=""}, {"Имя"="up0", "Группа"="up", "Наименование"="Переменная общего назначения 0", "Ед. изм"=0, "Список"="", "Адрес"=1792, "Описание"="Может использоваться для общих целей. Например, для запоминания длинны оси, приводимой в движение данным приводом и т.д.", "Мин"=-2147483647, "Макс"=2147483647, "Сервис"=FALSE, "Только чтение"=FALSE, "Разработка"=FALSE, "К-во бит"=32, "Шаг"=0, "Обработка"=FALSE, "Макрос"=""}, {"Имя"="up1", "Группа"="up", "Наименование"="Переменная общего назначения 1", "Ед. изм"=0, "Список"="", "Адрес"=1793, "Описание"="Может использоваться для общих целей. Например, для запоминания длинны оси, приводимой в движение данным приводом и т.д.", "Мин"=-2147483647, "Макс"=2147483647, "Сервис"=FALSE, "Только чтение"=FALSE, "Разработка"=FALSE, "К-во бит"=32, "Шаг"=0, "Обработка"=FALSE, "Макрос"=""}, {"Имя"="up2", "Группа"="up", "Наименование"="Переменная общего назначения 2", "Ед. изм"=0, "Список"="", "Адрес"=1794, "Описание"="Может использоваться для общих целей. Например, для запоминания длинны оси, приводимой в движение данным приводом и т.д.", "Мин"=-2147483647, "Макс"=2147483647, "Сервис"=FALSE, "Только чтение"=FALSE, "Разработка"=FALSE, "К-во бит"=32, "Шаг"=0, "Обработка"=FALSE, "Макрос"=""}, {"Имя"="up3", "Группа"="up", "Наименование"="Переменная общего назначения 3", "Ед. изм"=0, "Список"="", "Адрес"=1795, "Описание"="Может использоваться для общих целей. Например, для запоминания длинны оси, приводимой в движение данным приводом и т.д.", "Мин"=-2147483647, "Макс"=2147483647, "Сервис"=FALSE, "Только чтение"=FALSE, "Разработка"=FALSE, "К-во бит"=32, "Шаг"=0, "Обработка"=FALSE, "Макрос"=""}, {"Имя"="up4", "Группа"="up", "Наименование"="Переменная общего назначения 4", "Ед. изм"=0, "Список"="", "Адрес"=1796, "Описание"="Может использоваться для общих целей. Например, для запоминания длинны оси, приводимой в движение данным приводом и т.д.", "Мин"=-2147483647, "Макс"=2147483647, "Сервис"=FALSE, "Только чтение"=FALSE, "Разработка"=FALSE, "К-во бит"=32, "Шаг"=0, "Обработка"=FALSE, "Макрос"=""}, {"Имя"="up5", "Группа"="up", "Наименование"="Переменная общего назначения 5", "Ед. изм"=0, "Список"="", "Адрес"=1797, "Описание"="Может использоваться для общих целей. Например, для запоминания длинны оси, приводимой в движение данным приводом и т.д.", "Мин"=-2147483647, "Макс"=2147483647, "Сервис"=FALSE, "Только чтение"=FALSE, "Разработка"=FALSE, "К-во бит"=32, "Шаг"=0, "Обработка"=FALSE, "Макрос"=""}, {"Имя"="up6", "Группа"="up", "Наименование"="Переменная общего назначения 6", "Ед. изм"=0, "Список"="", "Адрес"=1798, "Описание"="Может использоваться для общих целей. Например, для запоминания длинны оси, приводимой в движение данным приводом и т.д.", "Мин"=-2147483647, "Макс"=2147483647, "Сервис"=FALSE, "Только чтение"=FALSE, "Разработка"=FALSE, "К-во бит"=32, "Шаг"=0, "Обработка"=FALSE, "Макрос"=""}, {"Имя"="up7", "Группа"="up", "Наименование"="Переменная общего назначения 7", "Ед. изм"=0, "Список"="", "Адрес"=1799, "Описание"="Может использоваться для общих целей. Например, для запоминания длинны оси, приводимой в движение данным приводом и т.д.", "Мин"=-2147483647, "Макс"=2147483647, "Сервис"=FALSE, "Только чтение"=FALSE, "Разработка"=FALSE, "К-во бит"=32, "Шаг"=0, "Обработка"=FALSE, "Макрос"=""}, {"Имя"="st4", "Группа"="st", "Наименование"="Тип привода", "Ед. изм"=0, "Список"="1:СПШ10-23xx\n2:СПШ20-23xx\\1000Z\n4:СПШ20-23xx\\2000Z\n64:СПШ10-34xx\n128:СПШ20-34xx\\2000Z\n4096:СПШ20-34xx\\1000Z\n8192:СПС25-80007\n8193:СПС25-80016\n8194:СПС25-80025\n8195:СПС25-1100075\n8196:СПС30-хххх\n\r\n", "Адрес"=70, "Описание"="", "Мин"=1, "Макс"=65535, "Сервис"=FALSE, "Только чтение"=FALSE, "Разработка"=FALSE, "К-во бит"=16, "Шаг"=0, "Обработка"=FALSE, "Макрос"=""}, {"Имя"="st5", "Группа"="st", "Наименование"="Z метка", "Ед. изм"=0, "Список"="0:Нет\n1:Да\n\r\n", "Адрес"=71, "Описание"="Наличие или отсутствие у датчика позиции канала нуливой метки", "Мин"=0, "Макс"=1, "Сервис"=FALSE, "Только чтение"=FALSE, "Разработка"=FALSE, "К-во бит"=16, "Шаг"=0, "Обработка"=FALSE, "Макрос"=""}, {"Имя"="cp6", "Группа"="cp", "Наименование"="Вырабатываемый момент", "Ед. изм"=0, "Список"="100:100%\n75:75%\n50:50%\n25:25%\n\r\n", "Адрес"=72, "Описание"="Параметр позволяет ограничить развиваемый момент", "Мин"=25, "Макс"=100, "Сервис"=FALSE, "Только чтение"=FALSE, "Разработка"=TRUE, "К-во бит"=16, "Шаг"=0, "Обработка"=FALSE, "Макрос"=""}, {"Имя"="ep3", "Группа"="ep", "Наименование"="Ток поиска фазы", "Ед. изм"=1, "Список"="", "Адрес"=81, "Описание"="Определяет уровень тока, который устанавливается при поиске фазы. Ток задается в дискретах.", "Мин"=0, "Макс"=32000, "Сервис"=FALSE, "Только чтение"=FALSE, "Разработка"=FALSE, "К-во бит"=16, "Шаг"=1, "Обработка"=FALSE, "Макрос"=""}, {"Имя"="ep4", "Группа"="ep", "Наименование"="Время поиска фазы", "Ед. изм"=1, "Список"="", "Адрес"=82, "Описание"="Определяет время, в течение которого будет удерживаться ток ep3 при поиске фазы.", "Мин"=0, "Макс"=32000, "Сервис"=FALSE, "Только чтение"=FALSE, "Разработка"=FALSE, "К-во бит"=16, "Шаг"=1, "Обработка"=FALSE, "Макрос"=""}, {"Имя"="ep5", "Группа"="ep", "Наименование"="Максимальная температура", "Ед. изм"=7, "Список"="", "Адрес"=84, "Описание"="Указывает максимальную допустимую температуру внутри корпуса", "Мин"=25, "Макс"=85, "Сервис"=FALSE, "Только чтение"=FALSE, "Разработка"=FALSE, "К-во бит"=16, "Шаг"=1, "Обработка"=FALSE, "Макрос"=""}, {"Имя"="cp7", "Группа"="cp", "Наименование"="Модуляция ШИМ сигнала", "Ед. изм"=0, "Список"="0:Выключена\n1:Включена\n\r\n", "Адрес"=83, "Описание"="Разрешает/запрещает подачу силового напряжения на обмотки двигателя", "Мин"=0, "Макс"=1, "Сервис"=FALSE, "Только чтение"=FALSE, "Разработка"=FALSE, "К-во бит"=16, "Шаг"=0, "Обработка"=FALSE, "Макрос"=""}, {"Имя"="ep6", "Группа"="ep", "Наименование"="Период поиска фазы", "Ед. изм"=0, "Список"="0:Однопериодный\n1:1\n2:2\n3:3\n\r\n", "Адрес"=86, "Описание"="Один из трех периодов, во время которого привод может выполнять поиск фазы. В результате удается избежать перегрузки источника питания и выполнить корректный поиск фазы в приводах, между которыми имеется жесткая механическая связь.", "Мин"=0, "Макс"=3, "Сервис"=FALSE, "Только чтение"=FALSE, "Разработка"=FALSE, "К-во бит"=16, "Шаг"=1, "Обработка"=FALSE, "Макрос"=""}, {"Имя"="up8", "Группа"="up", "Наименование"="X", "Ед. изм"=0, "Список"="", "Адрес"=1800, "Описание"="Переменная, используемая в ПЛК", "Мин"=-2147483647, "Макс"=2147483647, "Сервис"=FALSE, "Только чтение"=FALSE, "Разработка"=FALSE, "К-во бит"=32, "Шаг"=1, "Обработка"=FALSE, "Макрос"=""}, {"Имя"="up9", "Группа"="up", "Наименование"="Y", "Ед. изм"=0, "Список"="", "Адрес"=1801, "Описание"="Переменная, используемая в ПЛК", "Мин"=-2147483647, "Макс"=2147483647, "Сервис"=FALSE, "Только чтение"=FALSE, "Разработка"=FALSE, "К-во бит"=32, "Шаг"=1, "Обработка"=FALSE, "Макрос"=""}, {"Имя"="up10", "Группа"="up", "Наименование"="Z", "Ед. изм"=0, "Список"="", "Адрес"=1802, "Описание"="Переменная, используемая в ПЛК", "Мин"=-2147483647, "Макс"=2147483647, "Сервис"=FALSE, "Только чтение"=FALSE, "Разработка"=FALSE, "К-во бит"=32, "Шаг"=1, "Обработка"=FALSE, "Макрос"=""}, {"Имя"="up11", "Группа"="up", "Наименование"="EEPROM массив", "Ед. изм"=0, "Список"="", "Адрес"=1803, "Описание"="User EEPROM massive", "Мин"=-2147483647, "Макс"=2147483647, "Сервис"=FALSE, "Только чтение"=FALSE, "Разработка"=TRUE, "К-во бит"=32, "Шаг"=1, "Обработка"=FALSE, "Макрос"=""}, {"Имя"="up12", "Группа"="up", "Наименование"="EEPROM массив метаданных", "Ед. изм"=0, "Список"="", "Адрес"=1804, "Описание"="Metadata massive of params of motor", "Мин"=-2147483647, "Макс"=2147483647, "Сервис"=FALSE, "Только чтение"=FALSE, "Разработка"=TRUE, "К-во бит"=32, "Шаг"=1, "Обработка"=FALSE, "Макрос"=""}, {"Имя"="dd22", "Группа"="dd", "Наименование"="Максимальное отклонение от траектории", "Ед. изм"=1, "Список"="", "Адрес"=1056, "Описание"="Определяет максимальную ошибку контура позиции зафиксированную при прохождении траектории.", "Мин"=0, "Макс"=65535, "Сервис"=FALSE, "Только чтение"=FALSE, "Разработка"=FALSE, "К-во бит"=16, "Шаг"=0, "Обработка"=FALSE, "Макрос"=""}, {"Имя"="ip13", "Группа"="ip", "Наименование"="Ограничитель левый", "Ед. изм"=6, "Список"="", "Адрес"=87, "Описание"="Программный ограничитель позиции,  при достижении которой привод останавливается и воспринимает команду управления только в противоположную сторону.", "Мин"=-2147483647, "Макс"=2147483647, "Сервис"=FALSE, "Только чтение"=FALSE, "Разработка"=FALSE, "К-во бит"=32, "Шаг"=0, "Обработка"=FALSE, "Макрос"=""}, {"Имя"="ip14", "Группа"="ip", "Наименование"="Ограничитель правый", "Ед. изм"=6, "Список"="", "Адрес"=88, "Описание"="Программный ограничитель позиции,  при достижении которой привод останавливается и воспринимает команду управления только в противоположную сторону.", "Мин"=-2147483647, "Макс"=2147483647, "Сервис"=FALSE, "Только чтение"=FALSE, "Разработка"=FALSE, "К-во бит"=32, "Шаг"=0, "Обработка"=FALSE, "Макрос"=""}, {"Имя"="dd23", "Группа"="dd", "Наименование"="Статус G декодера", "Ед. изм"=0, "Список"="0:Останов\n1:Начало\n2:Отработка\n3:Ожидание подтверждений\n4:Ошибка\n5:Выход в нуль\r\n", "Адрес"=1057, "Описание"="", "Мин"=0, "Макс"=5, "Сервис"=FALSE, "Только чтение"=TRUE, "Разработка"=TRUE, "К-во бит"=16, "Шаг"=0, "Обработка"=FALSE, "Макрос"=""}, {"Имя"="dd24", "Группа"="dd", "Наименование"="Текущий кадр G декодера", "Ед. изм"=0, "Список"="", "Адрес"=1058, "Описание"="", "Мин"=0, "Макс"=65535, "Сервис"=FALSE, "Только чтение"=TRUE, "Разработка"=TRUE, "К-во бит"=16, "Шаг"=0, "Обработка"=FALSE, "Макрос"=""}, {"Имя"="ip15", "Группа"="ip", "Наименование"="Скорость обмена по шине CAN", "Ед. изм"=0, "Список"="500:500 кБит/сек\n1000:1000 кБит/сек\n\r\n", "Адрес"=89, "Описание"="Определяет скорость обмена по шине CAN. При этом допустимая скорость определяется дальностью линии связи. На скорость 1000кБит максимальная дальность 60м, 500кБит - 120м", "Мин"=50, "Макс"=1000, "Сервис"=FALSE, "Только чтение"=FALSE, "Разработка"=FALSE, "К-во бит"=16, "Шаг"=0, "Обработка"=FALSE, "Макрос"=""}, {"Имя"="cp8", "Группа"="cp", "Наименование"="Частота ШИМ сигнала", "Ед. изм"=12, "Список"="2500:40кГц\n5000:20кГц\n6250:16кГц\n12500:8кГц\n25000:4кГц\n\r\n", "Адрес"=96, "Описание"="Определяет частоту ШИМ сигнала и частоту работы контура тока. Влияет на КПД силовой части привода, а также качество работы контура тока. Для приводов серии СПШ частота всегда 40кГц. Влияет на параметр cp4.", "Мин"=-65535, "Макс"=65535, "Сервис"=FALSE, "Только чтение"=FALSE, "Разработка"=FALSE, "К-во бит"=16, "Шаг"=0, "Обработка"=FALSE, "Макрос"=""}, {"Имя"="ip16", "Группа"="ip", "Наименование"="USB2CAN конвертор", "Ед. изм"=0, "Список"="0:Выкл\n2:Вкл\n\r\n", "Адрес"=97, "Описание"="Данная функция предназначена для облегчения подключения к группе приводов СПШ/СПС, которые объединены в рамках системы в одну сеть CAN. Чтобы работать со всеми приводами сети достаточно подключиться только к одному приводу по USB.", "Мин"=0, "Макс"=2, "Сервис"=FALSE, "Только чтение"=FALSE, "Разработка"=FALSE, "К-во бит"=16, "Шаг"=0, "Обработка"=FALSE, "Макрос"=""}, {"Имя"="up13", "Группа"="up", "Наименование"="Значение текущего элемента EEPROM массива", "Ед. изм"=0, "Список"="", "Адрес"=1805, "Описание"="Отображает значение текущего элемента массива энергонезависимой памяти данных общего назначения.", "Мин"=-2147483647, "Макс"=2147483647, "Сервис"=FALSE, "Только чтение"=FALSE, "Разработка"=FALSE, "К-во бит"=32, "Шаг"=1, "Обработка"=FALSE, "Макрос"=""}, {"Имя"="up14", "Группа"="up", "Наименование"="Индекс текущего элемента EEPROM массива", "Ед. изм"=0, "Список"="", "Адрес"=1806, "Описание"="Отображает индекс текущего элемента массива энергонезависимой памяти данных общего назначения.", "Мин"=-2147483647, "Макс"=2147483647, "Сервис"=FALSE, "Только чтение"=FALSE, "Разработка"=FALSE, "К-во бит"=32, "Шаг"=1, "Обработка"=FALSE, "Макрос"=""}, {"Имя"="up15", "Группа"="up", "Наименование"="Значение счетчика импульсов", "Ед. изм"=0, "Список"="", "Адрес"=1807, "Описание"="Отображает значение счетчика импульсов, которые приходят на порты IN0, IN1, по протоколу Step\\Dir или по квадратурному протоколу. Счетчик активизирован только при выборе соответствующего протокола.", "Мин"=-2147483647, "Макс"=2147483647, "Сервис"=FALSE, "Только чтение"=FALSE, "Разработка"=FALSE, "К-во бит"=32, "Шаг"=1, "Обработка"=FALSE, "Макрос"=""}, {"Имя"="up16", "Группа"="up", "Наименование"="Среднее значение заданного тока", "Ед. изм"=0, "Список"="", "Адрес"=1808, "Описание"="Величина пропорциональна вырабатываемому приводом моменту, используется в программах для определения развиваемого момента.", "Мин"=-65535, "Макс"=65535, "Сервис"=FALSE, "Только чтение"=TRUE, "Разработка"=FALSE, "К-во бит"=16, "Шаг"=1, "Обработка"=FALSE, "Макрос"=""}, {"Имя"="ip17", "Группа"="ip", "Наименование"="Таймаут передачи синхронизации слейву", "Ед. изм"=9, "Список"="", "Адрес"=2048, "Описание"="Временной интервал, в течение которого мастер обязан передать синхронизацию слейву. По истечении этого времени параметр ip10 будет установлен в значение 1 или 2.", "Мин"=0, "Макс"=10000, "Сервис"=FALSE, "Только чтение"=FALSE, "Разработка"=FALSE, "К-во бит"=16, "Шаг"=25, "Обработка"=FALSE, "Макрос"=""}, {"Имя"="ip18", "Группа"="ip", "Наименование"="Таймаут передачи подтверждения мастеру от слейва", "Ед. изм"=9, "Список"="", "Адрес"=2049, "Описание"="Временной интервал, в течение которого слейв обязан передать подтверждение на команду синхронизации мастеру. По истечении этого времени параметр ip10 будет установлен в значение 3.", "Мин"=0, "Макс"=10000, "Сервис"=FALSE, "Только чтение"=FALSE, "Разработка"=FALSE, "К-во бит"=16, "Шаг"=25, "Обработка"=FALSE, "Макрос"=""}, {"Имя"="st6", "Группа"="st", "Наименование"="Нулевой сектор сигналов UVW", "Ед. изм"=0, "Список"="1:1\n2:2\n3:3\n4:4\n5:5\n6:6\n170:Выполнить инициализацию\n85:Не использовать UVW треки\n\r\n", "Адрес"=2050, "Описание"="Определяет сектор датчика UVW, в котором находится нуль двигателя. Если установить значение \"Выполнить инициализацию\", то при следующем запуске автоматически будет выполнена операция поиска сектора и смещения внутри сектора", "Мин"=0, "Макс"=170, "Сервис"=FALSE, "Только чтение"=FALSE, "Разработка"=FALSE, "К-во бит"=16, "Шаг"=0, "Обработка"=FALSE, "Макрос"=""}, {"Имя"="st7", "Группа"="st", "Наименование"="Сдвиг нуля внутри сектора сигналов UVW", "Ед. изм"=0, "Список"="", "Адрес"=2052, "Описание"="Определяет смещение внутри сектора датчика UVW, в котором находится нуль двигателя. Если установить значение \"Выполнить инициализацию\", то при следующем запуске автоматически будет выполнена операция поиска сектора и смещения внутри сектора", "Мин"=0, "Макс"=80000, "Сервис"=FALSE, "Только чтение"=FALSE, "Разработка"=FALSE, "К-во бит"=16, "Шаг"=0, "Обработка"=FALSE, "Макрос"=""}, {"Имя"="io0", "Группа"="io", "Наименование"="Порт ввода 0", "Ед. изм"=0, "Список"="", "Адрес"=2053, "Описание"="Значение порта ввода 0", "Мин"=0, "Макс"=1, "Сервис"=FALSE, "Только чтение"=FALSE, "Разработка"=FALSE, "К-во бит"=16, "Шаг"=0, "Обработка"=FALSE, "Макрос"=""}, {"Имя"="io1", "Группа"="io", "Наименование"="Порт ввода 1", "Ед. изм"=0, "Список"="", "Адрес"=2054, "Описание"="Значение порта ввода 1", "Мин"=0, "Макс"=1, "Сервис"=FALSE, "Только чтение"=FALSE, "Разработка"=FALSE, "К-во бит"=16, "Шаг"=0, "Обработка"=FALSE, "Макрос"=""}, {"Имя"="io2", "Группа"="io", "Наименование"="Порт ввода 2", "Ед. изм"=0, "Список"="", "Адрес"=2055, "Описание"="Значение порта ввода 2", "Мин"=0, "Макс"=1, "Сервис"=FALSE, "Только чтение"=FALSE, "Разработка"=FALSE, "К-во бит"=16, "Шаг"=0, "Обработка"=FALSE, "Макрос"=""}, {"Имя"="io3", "Группа"="io", "Наименование"="Порт ввода 3", "Ед. изм"=0, "Список"="", "Адрес"=2056, "Описание"="Значение порта ввода 3", "Мин"=0, "Макс"=1, "Сервис"=FALSE, "Только чтение"=FALSE, "Разработка"=FALSE, "К-во бит"=16, "Шаг"=0, "Обработка"=FALSE, "Макрос"=""}, {"Имя"="io4", "Группа"="io", "Наименование"="Порт вывода 0", "Ед. изм"=0, "Список"="", "Адрес"=2057, "Описание"="Значение порта вывода 0", "Мин"=0, "Макс"=1, "Сервис"=FALSE, "Только чтение"=FALSE, "Разработка"=FALSE, "К-во бит"=16, "Шаг"=0, "Обработка"=FALSE, "Макрос"=""}, {"Имя"="io5", "Группа"="io", "Наименование"="Порт вывода 1", "Ед. изм"=0, "Список"="", "Адрес"=2058, "Описание"="Значение порта вывода 1", "Мин"=0, "Макс"=1, "Сервис"=FALSE, "Только чтение"=FALSE, "Разработка"=FALSE, "К-во бит"=16, "Шаг"=0, "Обработка"=FALSE, "Макрос"=""}, {"Имя"="io6", "Группа"="io", "Наименование"="PWM0", "Ед. изм"=0, "Список"="", "Адрес"=2059, "Описание"="Скваженность ШИМ сигнала, выводимого на порт вывода 0. Порт необходимо соответствующим образом настроить с помощью параметра: Режим работы порта вывода.", "Мин"=0, "Макс"=160, "Сервис"=FALSE, "Только чтение"=FALSE, "Разработка"=FALSE, "К-во бит"=16, "Шаг"=1, "Обработка"=FALSE, "Макрос"=""}, {"Имя"="io7", "Группа"="io", "Наименование"="PWM1", "Ед. изм"=0, "Список"="", "Адрес"=2060, "Описание"="Скваженность ШИМ сигнала, выводимого на порт вывода 1. Порт необходимо соответствующим образом настроить с помощью параметра: Режим работы порта вывода.", "Мин"=0, "Макс"=160, "Сервис"=FALSE, "Только чтение"=FALSE, "Разработка"=FALSE, "К-во бит"=16, "Шаг"=1, "Обработка"=FALSE, "Макрос"=""}, {"Имя"="io8", "Группа"="io", "Наименование"="Режим порта ввода 0", "Ед. изм"=0, "Список"="0:Порт ввода общего назначения\n1:Порт ввода в режиме квадратурного счетчика\n2:Порт ввода в режиме счетчика Step/dir\n\r\n", "Адрес"=2061, "Описание"="Определяет режим работы порта ввода.", "Мин"=0, "Макс"=3, "Сервис"=FALSE, "Только чтение"=FALSE, "Разработка"=FALSE, "К-во бит"=16, "Шаг"=1, "Обработка"=FALSE, "Макрос"=""}, {"Имя"="io9", "Группа"="io", "Наименование"="Режим порта ввода 1", "Ед. изм"=0, "Список"="0:Порт ввода общего назначения\n1:Порт ввода в режиме квадратурного счетчика\n2:Порт ввода в режиме счетчика Step/dir\n\r\n", "Адрес"=2062, "Описание"="Определяет режим работы порта ввода.", "Мин"=0, "Макс"=3, "Сервис"=FALSE, "Только чтение"=FALSE, "Разработка"=FALSE, "К-во бит"=16, "Шаг"=1, "Обработка"=FALSE, "Макрос"=""}, {"Имя"="io10", "Группа"="io", "Наименование"="Режим порта ввода 2", "Ед. изм"=0, "Список"="0:Порт ввода общего назначения\n1:Порт ввода в режиме квадратурного счетчика\n2:Порт ввода в режиме счетчика Step/dir\n\r\n", "Адрес"=2063, "Описание"="Определяет режим работы порта ввода.", "Мин"=0, "Макс"=3, "Сервис"=FALSE, "Только чтение"=FALSE, "Разработка"=FALSE, "К-во бит"=16, "Шаг"=1, "Обработка"=FALSE, "Макрос"=""}, {"Имя"="io11", "Группа"="io", "Наименование"="Режим порта ввода 3", "Ед. изм"=0, "Список"="0:Порт ввода общего назначения\n1:Порт ввода в режиме квадратурного счетчика\n2:Порт ввода в режиме счетчика Step/dir\n\r\n", "Адрес"=2064, "Описание"="Определяет режим работы порта ввода.", "Мин"=0, "Макс"=3, "Сервис"=FALSE, "Только чтение"=FALSE, "Разработка"=FALSE, "К-во бит"=16, "Шаг"=1, "Обработка"=FALSE, "Макрос"=""}, {"Имя"="io12", "Группа"="io", "Наименование"="Режим порта вывода 0", "Ед. изм"=0, "Список"="0:Порт вывода общего назначения\n1:Порт вывода в режиме ШИМ\n\r\n", "Адрес"=2065, "Описание"="Определяет режим работы порта вывода.", "Мин"=0, "Макс"=3, "Сервис"=FALSE, "Только чтение"=FALSE, "Разработка"=FALSE, "К-во бит"=16, "Шаг"=1, "Обработка"=FALSE, "Макрос"=""}, {"Имя"="io13", "Группа"="io", "Наименование"="Режим порта вывода 1", "Ед. изм"=0, "Список"="0:Порт вывода общего назначения\n1:Порт вывода в режиме ШИМ\n\r\n", "Адрес"=2066, "Описание"="Определяет режим работы порта вывода.", "Мин"=0, "Макс"=3, "Сервис"=FALSE, "Только чтение"=FALSE, "Разработка"=FALSE, "К-во бит"=16, "Шаг"=1, "Обработка"=FALSE, "Макрос"=""}, {"Имя"="io14", "Группа"="io", "Наименование"="Счетчик импульсов", "Ед. изм"=0, "Список"="", "Адрес"=1807, "Описание"="Аппаратный счетчик импульсов,  которые приходят на входы In0 и In1. При этом порты должны быть настроены на соответствующий интерфейс (см. параметры io8 и io9).", "Мин"=-2147483647, "Макс"=2147483647, "Сервис"=FALSE, "Только чтение"=TRUE, "Разработка"=FALSE, "К-во бит"=32, "Шаг"=1, "Обработка"=FALSE, "Макрос"=""}, {"Имя"="dd25", "Группа"="dd", "Наименование"="UVW треки", "Ед. изм"=0, "Список"="", "Адрес"=1059, "Описание"="Сигнал, считанный с UVW треков энкодера", "Мин"=0, "Макс"=16, "Сервис"=FALSE, "Только чтение"=TRUE, "Разработка"=FALSE, "К-во бит"=16, "Шаг"=0, "Обработка"=FALSE, "Макрос"=""}, {"Имя"="st8", "Группа"="st", "Наименование"="Тип энкодера", "Ед. изм"=0, "Список"="0:Инкрементальный\n1:Абсолютный\n\r\n", "Адрес"=98, "Описание"="", "Мин"=0, "Макс"=1, "Сервис"=FALSE, "Только чтение"=FALSE, "Разработка"=FALSE, "К-во бит"=32, "Шаг"=1, "Обработка"=FALSE, "Макрос"=""}, {"Имя"="vp17", "Группа"="vp", "Наименование"="Рывок", "Ед. изм"=0, "Список"="", "Адрес"=99, "Описание"="Ограничивает вторую производную скорости. Параметр вступает в силу только при установки vp9 в значение 4", "Мин"=1, "Макс"=21470, "Сервис"=TRUE, "Только чтение"=FALSE, "Разработка"=FALSE, "К-во бит"=32, "Шаг"=10, "Обработка"=FALSE, "Макрос"=""}, {"Имя"="cp9", "Группа"="cp", "Наименование"="Допустимая перегрузка", "Ед. изм"=13, "Список"="", "Адрес"=2068, "Описание"="Ограничение выделяемой мощности обмотками двигателя. Предотвращает повреждения обмоток. Реализует защитную функцию I2t", "Мин"=0, "Макс"=350, "Сервис"=TRUE, "Только чтение"=FALSE, "Разработка"=FALSE, "К-во бит"=32, "Шаг"=16, "Обработка"=FALSE, "Макрос"=""}, {"Имя"="cp10", "Группа"="cp", "Наименование"="Номинальный ток", "Ед. изм"=5, "Список"="", "Адрес"=2069, "Описание"="", "Мин"=0, "Макс"=850, "Сервис"=TRUE, "Только чтение"=FALSE, "Разработка"=FALSE, "К-во бит"=32, "Шаг"=16, "Обработка"=TRUE, "Макрос"="macros cp10\n  ON_READ\n  READ cp3\n  cp3=cp3*5/2047\n  RETURN cp3\n  ON_WRITE\n  cp3=val*66\n  WRITE cp3\nend"}, {"Имя"="dd26", "Группа"="dd", "Наименование"="Текущая перегрузка", "Ед. изм"=13, "Список"="", "Адрес"=1060, "Описание"="Накомпленнае мощность, превышающая номинальные характеристики двигателя", "Мин"=0, "Макс"=100, "Сервис"=TRUE, "Только чтение"=TRUE, "Разработка"=FALSE, "К-во бит"=32, "Шаг"=16, "Обработка"=FALSE, "Макрос"=""}, {"Имя"="dd27", "Группа"="dd", "Наименование"="Ток в обмотке 3", "Ед. изм"=5, "Список"="", "Адрес"=1061, "Описание"="Показывает ток, протекающий в обмотке двигателя. Параметр действителен только для СПС.", "Мин"=-5, "Макс"=5, "Сервис"=FALSE, "Только чтение"=TRUE, "Разработка"=FALSE, "К-во бит"=16, "Шаг"=0, "Обработка"=TRUE, "Макрос"="macros dd27\n  ON_READ\n  READ dd1\n  dd1=dd1*5/2047\n  RETURN dd1\n  ON_WRITE\n  dd1=val*2047/5\n  WRITE dd1\nend"}, {"Имя"="dd28", "Группа"="dd", "Наименование"="Заданный ток в обмотке 3", "Ед. изм"=5, "Список"="", "Адрес"=1062, "Описание"="Заданный ток в обмотке 3. Действителен только для приводов серии СПС.", "Мин"=-2047, "Макс"=2047, "Сервис"=FALSE, "Только чтение"=FALSE, "Разработка"=FALSE, "К-во бит"=16, "Шаг"=0, "Обработка"=TRUE, "Макрос"="macros dd28\n  ON_READ\n  READ dd6\n  dd6=dd6/74\n  RETURN dd6\n  ON_WRITE\n  dd6=val*74\n  WRITE dd6\nend"}, {"Имя"="dd29", "Группа"="dd", "Наименование"="Ток потребления двигателя", "Ед. изм"=5, "Список"="", "Адрес"=1063, "Описание"="Параметр действителен только для СПС.", "Мин"=-5, "Макс"=5, "Сервис"=FALSE, "Только чтение"=TRUE, "Разработка"=FALSE, "К-во бит"=16, "Шаг"=0, "Обработка"=TRUE, "Макрос"="macros dd29\n  ON_READ\n  READ dd1\n  dd1=dd1/74\n  RETURN dd1\n  ON_WRITE\n  dd1=val*74\n  WRITE dd1\nend"}, {"Имя"="pd1", "Группа"="pd", "Наименование"="Зона нечувствительности", "Ед. изм"=0, "Список"="", "Адрес"=2561, "Описание"="Параметр настройки ПИД-регулятора", "Мин"=0, "Макс"=10000, "Сервис"=TRUE, "Только чтение"=FALSE, "Разработка"=FALSE, "К-во бит"=32, "Шаг"=12, "Обработка"=FALSE, "Макрос"=""}, {"Имя"="pd2", "Группа"="pd", "Наименование"="Максимальная ошибка", "Ед. изм"=0, "Список"="", "Адрес"=2562, "Описание"="Параметр настройки ПИД-регулятора", "Мин"=0, "Макс"=524287, "Сервис"=TRUE, "Только чтение"=FALSE, "Разработка"=FALSE, "К-во бит"=32, "Шаг"=12, "Обработка"=FALSE, "Макрос"=""}, {"Имя"="pd3", "Группа"="pd", "Наименование"="Пропорциональный коэффициент", "Ед. изм"=0, "Список"="", "Адрес"=2563, "Описание"="Параметр настройки ПИД-регулятора", "Мин"=0, "Макс"=10000, "Сервис"=TRUE, "Только чтение"=FALSE, "Разработка"=FALSE, "К-во бит"=32, "Шаг"=12, "Обработка"=FALSE, "Макрос"=""}, {"Имя"="pd4", "Группа"="pd", "Наименование"="Интегральный коэффициент", "Ед. изм"=0, "Список"="", "Адрес"=2564, "Описание"="Параметр настройки ПИД-регулятора", "Мин"=0, "Макс"=10000, "Сервис"=TRUE, "Только чтение"=FALSE, "Разработка"=FALSE, "К-во бит"=32, "Шаг"=12, "Обработка"=FALSE, "Макрос"=""}, {"Имя"="pd5", "Группа"="pd", "Наименование"="Дифференциальный коэффициент", "Ед. изм"=0, "Список"="", "Адрес"=2565, "Описание"="Параметр настройки ПИД-регулятора", "Мин"=0, "Макс"=10000, "Сервис"=TRUE, "Только чтение"=FALSE, "Разработка"=FALSE, "К-во бит"=32, "Шаг"=12, "Обработка"=FALSE, "Макрос"=""}, {"Имя"="pd6", "Группа"="pd", "Наименование"="Ограничение интегральной составляющей", "Ед. изм"=0, "Список"="", "Адрес"=2566, "Описание"="Параметр настройки ПИД-регулятора", "Мин"=0, "Макс"=100000, "Сервис"=TRUE, "Только чтение"=FALSE, "Разработка"=FALSE, "К-во бит"=32, "Шаг"=12, "Обработка"=FALSE, "Макрос"=""}, {"Имя"="pd7", "Группа"="pd", "Наименование"="Ограничение дифференциальной составляющей", "Ед. изм"=0, "Список"="", "Адрес"=2567, "Описание"="Параметр настройки ПИД-регулятора", "Мин"=0, "Макс"=100000, "Сервис"=TRUE, "Только чтение"=FALSE, "Разработка"=FALSE, "К-во бит"=32, "Шаг"=12, "Обработка"=FALSE, "Макрос"=""}, {"Имя"="pd8", "Группа"="pd", "Наименование"="Ограничение форсирующей составляющей 1го порядка", "Ед. изм"=0, "Список"="", "Адрес"=2568, "Описание"="Параметр настройки ПИД-регулятора", "Мин"=0, "Макс"=524287, "Сервис"=TRUE, "Только чтение"=FALSE, "Разработка"=FALSE, "К-во бит"=32, "Шаг"=12, "Обработка"=FALSE, "Макрос"=""}, {"Имя"="pd9", "Группа"="pd", "Наименование"="Ограничение форсирующей составляющей 2го порядка", "Ед. изм"=0, "Список"="", "Адрес"=2569, "Описание"="Параметр настройки ПИД-регулятора", "Мин"=0, "Макс"=524287, "Сервис"=TRUE, "Только чтение"=FALSE, "Разработка"=FALSE, "К-во бит"=32, "Шаг"=12, "Обработка"=FALSE, "Макрос"=""}, {"Имя"="pd10", "Группа"="pd", "Наименование"="Коэффициент форсирующей составляющей 0го порядка", "Ед. изм"=0, "Список"="", "Адрес"=2570, "Описание"="Параметр настройки ПИД-регулятора", "Мин"=0, "Макс"=10000, "Сервис"=TRUE, "Только чтение"=FALSE, "Разработка"=FALSE, "К-во бит"=32, "Шаг"=12, "Обработка"=FALSE, "Макрос"=""}, {"Имя"="pd11", "Группа"="pd", "Наименование"="Коэффициент форсирующей составляющей 1го порядка", "Ед. изм"=0, "Список"="", "Адрес"=2571, "Описание"="Параметр настройки ПИД-регулятора", "Мин"=0, "Макс"=10000, "Сервис"=TRUE, "Только чтение"=FALSE, "Разработка"=FALSE, "К-во бит"=32, "Шаг"=12, "Обработка"=FALSE, "Макрос"=""}, {"Имя"="pd12", "Группа"="pd", "Наименование"="Коэффициент форсирующей составляющей 2го порядка", "Ед. изм"=0, "Список"="", "Адрес"=2572, "Описание"="Параметр настройки ПИД-регулятора", "Мин"=0, "Макс"=10000, "Сервис"=TRUE, "Только чтение"=FALSE, "Разработка"=FALSE, "К-во бит"=32, "Шаг"=12, "Обработка"=FALSE, "Макрос"=""}, {"Имя"="pd13", "Группа"="pd", "Наименование"="Смещение сигнала управления", "Ед. изм"=0, "Список"="", "Адрес"=2573, "Описание"="Параметр настройки ПИД-регулятора", "Мин"=-524286, "Макс"=524287, "Сервис"=TRUE, "Только чтение"=FALSE, "Разработка"=FALSE, "К-во бит"=32, "Шаг"=12, "Обработка"=FALSE, "Макрос"=""}, {"Имя"="pd14", "Группа"="pd", "Наименование"="Ограничение выходного сигнала", "Ед. изм"=0, "Список"="", "Адрес"=2574, "Описание"="Параметр настройки ПИД-регулятора", "Мин"=0, "Макс"=524287, "Сервис"=TRUE, "Только чтение"=FALSE, "Разработка"=FALSE, "К-во бит"=32, "Шаг"=12, "Обработка"=FALSE, "Макрос"=""}, {"Имя"="pd15", "Группа"="pd", "Наименование"="Задание регулятора", "Ед. изм"=0, "Список"="", "Адрес"=2575, "Описание"="Параметр настройки ПИД-регулятора", "Мин"=-524286, "Макс"=524287, "Сервис"=TRUE, "Только чтение"=FALSE, "Разработка"=FALSE, "К-во бит"=32, "Шаг"=12, "Обработка"=FALSE, "Макрос"=""}, {"Имя"="pd16", "Группа"="pd", "Наименование"="Обратная связь", "Ед. изм"=0, "Список"="", "Адрес"=2576, "Описание"="Параметр настройки ПИД-регулятора", "Мин"=-524286, "Макс"=524287, "Сервис"=TRUE, "Только чтение"=TRUE, "Разработка"=FALSE, "К-во бит"=32, "Шаг"=12, "Обработка"=FALSE, "Макрос"=""}, {"Имя"="pd17", "Группа"="pd", "Наименование"="Ошибка", "Ед. изм"=0, "Список"="", "Адрес"=2577, "Описание"="Параметр настройки ПИД-регулятора", "Мин"=-524286, "Макс"=524287, "Сервис"=TRUE, "Только чтение"=TRUE, "Разработка"=FALSE, "К-во бит"=32, "Шаг"=12, "Обработка"=FALSE, "Макрос"=""}, {"Имя"="pp7", "Группа"="pp", "Наименование"="Ограничение форсирующей составляющей 1го порядка", "Ед. изм"=0, "Список"="", "Адрес"=2578, "Описание"="Параметр настройки ПИД-регулятора", "Мин"=0, "Макс"=524287, "Сервис"=TRUE, "Только чтение"=FALSE, "Разработка"=FALSE, "К-во бит"=32, "Шаг"=10, "Обработка"=FALSE, "Макрос"=""}, {"Имя"="pp8", "Группа"="pp", "Наименование"="Ограничение форсирующей составляющей 2го порядка", "Ед. изм"=0, "Список"="", "Адрес"=2579, "Описание"="Параметр настройки ПИД-регулятора", "Мин"=0, "Макс"=524287, "Сервис"=TRUE, "Только чтение"=FALSE, "Разработка"=FALSE, "К-во бит"=32, "Шаг"=10, "Обработка"=FALSE, "Макрос"=""}, {"Имя"="pp9", "Группа"="pp", "Наименование"="Коэффициент форсирующей составляющей 1го порядка", "Ед. изм"=0, "Список"="", "Адрес"=2580, "Описание"="Параметр настройки ПИД-регулятора", "Мин"=0, "Макс"=100000, "Сервис"=TRUE, "Только чтение"=FALSE, "Разработка"=FALSE, "К-во бит"=32, "Шаг"=10, "Обработка"=FALSE, "Макрос"=""}, {"Имя"="pp10", "Группа"="pp", "Наименование"="Коэффициент форсирующей составляющей 2го порядка", "Ед. изм"=0, "Список"="", "Адрес"=2581, "Описание"="Параметр настройки ПИД-регулятора", "Мин"=0, "Макс"=100000, "Сервис"=TRUE, "Только чтение"=FALSE, "Разработка"=FALSE, "К-во бит"=32, "Шаг"=10, "Обработка"=FALSE, "Макрос"=""}, {"Имя"="vp18", "Группа"="vp", "Наименование"="Зона нечувствительности входного сигнала", "Ед. изм"=0, "Список"="", "Адрес"=2582, "Описание"="Параметр настройки ПИ-регулятора контура скорости", "Мин"=0, "Макс"=60000, "Сервис"=TRUE, "Только чтение"=FALSE, "Разработка"=FALSE, "К-во бит"=32, "Шаг"=12, "Обработка"=FALSE, "Макрос"=""}, {"Имя"="vp19", "Группа"="vp", "Наименование"="Максимальная ошибка", "Ед. изм"=0, "Список"="", "Адрес"=2583, "Описание"="Параметр настройки ПИ-регулятора контура скорости", "Мин"=0, "Макс"=60000, "Сервис"=TRUE, "Только чтение"=FALSE, "Разработка"=FALSE, "К-во бит"=32, "Шаг"=12, "Обработка"=FALSE, "Макрос"=""}, {"Имя"="vp20", "Группа"="vp", "Наименование"="Ограничение форсирующей связи 1го порядка", "Ед. изм"=0, "Список"="", "Адрес"=2584, "Описание"="Параметр настройки ПИ-регулятора контура скорости", "Мин"=0, "Макс"=524287, "Сервис"=TRUE, "Только чтение"=FALSE, "Разработка"=FALSE, "К-во бит"=32, "Шаг"=12, "Обработка"=FALSE, "Макрос"=""}, {"Имя"="vp21", "Группа"="vp", "Наименование"="Ограничение форсирующей связи 2го порядка", "Ед. изм"=0, "Список"="", "Адрес"=2585, "Описание"="Параметр настройки ПИ-регулятора контура скорости", "Мин"=0, "Макс"=524287, "Сервис"=TRUE, "Только чтение"=FALSE, "Разработка"=FALSE, "К-во бит"=32, "Шаг"=12, "Обработка"=FALSE, "Макрос"=""}, {"Имя"="vp22", "Группа"="vp", "Наименование"="Коэффициент форсирующей связи 0го порядка", "Ед. изм"=0, "Список"="", "Адрес"=2586, "Описание"="Параметр настройки ПИ-регулятора контура скорости", "Мин"=0, "Макс"=60000, "Сервис"=TRUE, "Только чтение"=FALSE, "Разработка"=FALSE, "К-во бит"=32, "Шаг"=12, "Обработка"=FALSE, "Макрос"=""}, {"Имя"="vp23", "Группа"="vp", "Наименование"="Коэффициент форсирующей связи 1го порядка", "Ед. изм"=0, "Список"="", "Адрес"=2587, "Описание"="Параметр настройки ПИ-регулятора контура скорости", "Мин"=0, "Макс"=60000, "Сервис"=TRUE, "Только чтение"=FALSE, "Разработка"=FALSE, "К-во бит"=32, "Шаг"=12, "Обработка"=FALSE, "Макрос"=""}, {"Имя"="vp24", "Группа"="vp", "Наименование"="Коэффициент форсирующей связи 2го порядка", "Ед. изм"=0, "Список"="", "Адрес"=2588, "Описание"="Параметр настройки ПИ-регулятора контура скорости", "Мин"=0, "Макс"=60000, "Сервис"=TRUE, "Только чтение"=FALSE, "Разработка"=FALSE, "К-во бит"=32, "Шаг"=12, "Обработка"=FALSE, "Макрос"=""}, {"Имя"="st9", "Группа"="st", "Наименование"="Линейный энкодер", "Ед. изм"=0, "Список"="0:Нет\n1:Да\n\r\n", "Адрес"=2070, "Описание"="Если параметр установлен в Да, то будет использоваться внешний по отношению к приводу линейный энкодер для замыкания контура позиции. При этом контуры тока и скорости будут работать, по прежнему, от внутреннего энкодера.", "Мин"=0, "Макс"=1, "Сервис"=FALSE, "Только чтение"=FALSE, "Разработка"=FALSE, "К-во бит"=16, "Шаг"=0, "Обработка"=FALSE, "Макрос"=""}, {"Имя"="st10", "Группа"="st", "Наименование"="Разрешение линейного энкодера", "Ед. изм"=1, "Список"="", "Адрес"=2071, "Описание"="Разрешение линейного энкодера на оборот вала двигателя", "Мин"=-524286, "Макс"=524286, "Сервис"=TRUE, "Только чтение"=FALSE, "Разработка"=FALSE, "К-во бит"=32, "Шаг"=12, "Обработка"=FALSE, "Макрос"=""}, {"Имя"="dd30", "Группа"="dd", "Наименование"="Разница между внешним и внутренним энкодерами", "Ед. изм"=1, "Список"="", "Адрес"=1064, "Описание"="Разница между внешним и внутренним энкодерами с приведением к разрешению внутреннего", "Мин"=-524286, "Макс"=524286, "Сервис"=TRUE, "Только чтение"=TRUE, "Разработка"=FALSE, "К-во бит"=32, "Шаг"=12, "Обработка"=FALSE, "Макрос"=""}, {"Имя"="ss16", "Группа"="ss", "Наименование"="Счетчик потерь синхронизации", "Ед. изм"=0, "Список"="", "Адрес"=2072, "Описание"="Показывает сколько было потеряно команд SYNC=0x02 по шине CAN. Счетчик работает только, если выбран один из возможных режимов синхронизации.", "Мин"=0, "Макс"=65535, "Сервис"=FALSE, "Только чтение"=FALSE, "Разработка"=FALSE, "К-во бит"=16, "Шаг"=0, "Обработка"=FALSE, "Макрос"=""}, {"Имя"="ss17", "Группа"="ss", "Наименование"="Счетчик потерь команд управления", "Ед. изм"=0, "Список"="", "Адрес"=2073, "Описание"="Показывает сколько было потеряно команд CAN_POS_COM=0x08 по шине CAN. Счетчик работает только, если выбран один из возможных режимов синхронизации.", "Мин"=0, "Макс"=65535, "Сервис"=FALSE, "Только чтение"=FALSE, "Разработка"=FALSE, "К-во бит"=16, "Шаг"=0, "Обработка"=FALSE, "Макрос"=""}, {"Имя"="ss18", "Группа"="ss", "Наименование"="Счетчик получения неизвестных команд", "Ед. изм"=0, "Список"="", "Адрес"=2074, "Описание"="Показывает сколько было получено неизвестных команд по шине CAN, которые помешали прохождению команд управления. Счетчик работает только, если выбран один из возможных режимов синхронизации.", "Мин"=0, "Макс"=65535, "Сервис"=FALSE, "Только чтение"=FALSE, "Разработка"=FALSE, "К-во бит"=16, "Шаг"=0, "Обработка"=FALSE, "Макрос"=""}, {"Имя"="pd18", "Группа"="pd", "Наименование"="Коэффициент ФНЧ входного сигнала", "Ед. изм"=0, "Список"="", "Адрес"=2589, "Описание"="Параметр настройки ПИД-регулятора", "Мин"=0, "Макс"=1, "Сервис"=TRUE, "Только чтение"=FALSE, "Разработка"=FALSE, "К-во бит"=32, "Шаг"=12, "Обработка"=FALSE, "Макрос"=""}, {"Имя"="pd19", "Группа"="pd", "Наименование"="Коэффициент ФНЧ сигнала обратной связи", "Ед. изм"=0, "Список"="", "Адрес"=2590, "Описание"="Параметр настройки ПИД-регулятора", "Мин"=0, "Макс"=1, "Сервис"=TRUE, "Только чтение"=FALSE, "Разработка"=FALSE, "К-во бит"=32, "Шаг"=12, "Обработка"=FALSE, "Макрос"=""}, {"Имя"="ep7", "Группа"="ep", "Наименование"="Функция контроля зазора", "Ед. изм"=0, "Список"="0:ВЫКЛ\n90:ВКЛ\n\r\n", "Адрес"=2075, "Описание"="Включение данной автоматически запускает внутреннюю программу контроля расстояния между инструментом и обрабатываемым листом.", "Мин"=0, "Макс"=90, "Сервис"=FALSE, "Только чтение"=FALSE, "Разработка"=FALSE, "К-во бит"=16, "Шаг"=1, "Обработка"=FALSE, "Макрос"=""}, {"Имя"="pp11", "Группа"="pp", "Наименование"="Коэффициент микроинтерполяции", "Ед. изм"=0, "Список"="1:1\n2:2\n3:3\n4:4\n5:5\n\r\n", "Адрес"=2076, "Описание"="Коэффициент микроинтерполяции определяет кратность соотношения частот квантования СЧПУ и контура позиции привода. Коэффициент может принимать только значения 1, 2, 3, 4, 5. Если коэффициент равен 1, то частоты СЧПУ и привода равны.", "Мин"=1, "Макс"=5, "Сервис"=TRUE, "Только чтение"=FALSE, "Разработка"=FALSE, "К-во бит"=32, "Шаг"=10, "Обработка"=FALSE, "Макрос"=""}, {"Имя"="ip19", "Группа"="ip", "Наименование"="Данные CAN собщения 0", "Ед. изм"=0, "Список"="", "Адрес"=2077, "Описание"="4 младших байта последнего полученного CAN собщения", "Мин"=-2147483637, "Макс"=2147483646, "Сервис"=FALSE, "Только чтение"=FALSE, "Разработка"=FALSE, "К-во бит"=32, "Шаг"=0, "Обработка"=FALSE, "Макрос"=""}, {"Имя"="ip20", "Группа"="ip", "Наименование"="Данные CAN собщения 1", "Ед. изм"=0, "Список"="", "Адрес"=2078, "Описание"="4 старших байта последнего полученного CAN собщения", "Мин"=-2147483637, "Макс"=2147483646, "Сервис"=FALSE, "Только чтение"=FALSE, "Разработка"=FALSE, "К-во бит"=32, "Шаг"=0, "Обработка"=FALSE, "Макрос"=""}, {"Имя"="dd31", "Группа"="dd", "Наименование"="Смещение фазы ослабления поля", "Ед. изм"=0, "Список"="", "Адрес"=1065, "Описание"="", "Мин"=0, "Макс"=0, "Сервис"=FALSE, "Только чтение"=TRUE, "Разработка"=FALSE, "К-во бит"=16, "Шаг"=0, "Обработка"=FALSE, "Макрос"=""}, {"Имя"="vp25", "Группа"="vp", "Наименование"="Коэффициент ФНЧ входного сигнала", "Ед. изм"=0, "Список"="", "Адрес"=2079, "Описание"="Коэффициент ФНЧ входного сигнала контура скорости", "Мин"=0, "Макс"=1, "Сервис"=TRUE, "Только чтение"=FALSE, "Разработка"=FALSE, "К-во бит"=32, "Шаг"=12, "Обработка"=FALSE, "Макрос"=""}, {"Имя"="vp26", "Группа"="vp", "Наименование"="Коэффициент ФНЧ сигнала обратной связи", "Ед. изм"=0, "Список"="", "Адрес"=2080, "Описание"="Коэффициент ФНЧ сигнала обратной связи контура скорости", "Мин"=0, "Макс"=1, "Сервис"=TRUE, "Только чтение"=FALSE, "Разработка"=FALSE, "К-во бит"=32, "Шаг"=12, "Обработка"=FALSE, "Макрос"=""}, {"Имя"="up17", "Группа"="up", "Наименование"="Переменная общего назначения 8", "Ед. изм"=0, "Список"="", "Адрес"=1809, "Описание"="Может использоваться для общих целей. ВНИМАНИЕ! Данная переменная не записывается в энергонезависимую память.", "Мин"=-2147483647, "Макс"=2147483647, "Сервис"=FALSE, "Только чтение"=FALSE, "Разработка"=FALSE, "К-во бит"=32, "Шаг"=0, "Обработка"=FALSE, "Макрос"=""}, {"Имя"="up18", "Группа"="up", "Наименование"="Переменная общего назначения 9", "Ед. изм"=0, "Список"="", "Адрес"=1810, "Описание"="Может использоваться для общих целей. ВНИМАНИЕ! Данная переменная не записывается в энергонезависимую память.", "Мин"=-2147483647, "Макс"=2147483647, "Сервис"=FALSE, "Только чтение"=FALSE, "Разработка"=FALSE, "К-во бит"=32, "Шаг"=0, "Обработка"=FALSE, "Макрос"=""}, {"Имя"="up19", "Группа"="up", "Наименование"="Переменная общего назначения 10", "Ед. изм"=0, "Список"="", "Адрес"=1811, "Описание"="", "Мин"=-2147483647, "Макс"=2147483647, "Сервис"=FALSE, "Только чтение"=FALSE, "Разработка"=FALSE, "К-во бит"=32, "Шаг"=0, "Обработка"=FALSE, "Макрос"=""}, {"Имя"="up20", "Группа"="up", "Наименование"="Переменная общего назначения 11", "Ед. изм"=0, "Список"="", "Адрес"=1812, "Описание"="", "Мин"=-2147483647, "Макс"=2147483647, "Сервис"=FALSE, "Только чтение"=FALSE, "Разработка"=FALSE, "К-во бит"=32, "Шаг"=0, "Обработка"=FALSE, "Макрос"=""}, {"Имя"="up21", "Группа"="up", "Наименование"="Переменная общего назначения 12", "Ед. изм"=0, "Список"="", "Адрес"=1813, "Описание"="Может использоваться для общих целей. ВНИМАНИЕ! Данная переменная не записывается в энергонезависимую память.", "Мин"=-2147483647, "Макс"=2147483647, "Сервис"=FALSE, "Только чтение"=FALSE, "Разработка"=FALSE, "К-во бит"=32, "Шаг"=0, "Обработка"=FALSE, "Макрос"=""}, {"Имя"="up22", "Группа"="up", "Наименование"="Переменная общего назначения 13", "Ед. изм"=0, "Список"="", "Адрес"=1814, "Описание"="Может использоваться для общих целей. ВНИМАНИЕ! Данная переменная не записывается в энергонезависимую память.", "Мин"=-2147483647, "Макс"=2147483647, "Сервис"=FALSE, "Только чтение"=FALSE, "Разработка"=FALSE, "К-во бит"=32, "Шаг"=0, "Обработка"=FALSE, "Макрос"=""}, {"Имя"="up23", "Группа"="up", "Наименование"="Переменная общего назначения  14", "Ед. изм"=0, "Список"="", "Адрес"=1815, "Описание"="Может использоваться для общих целей. ВНИМАНИЕ! Данная переменная не записывается в энергонезависимую память.", "Мин"=-2147483647, "Макс"=2147483647, "Сервис"=FALSE, "Только чтение"=FALSE, "Разработка"=FALSE, "К-во бит"=32, "Шаг"=0, "Обработка"=FALSE, "Макрос"=""}, {"Имя"="up24", "Группа"="up", "Наименование"="Переменная общего назначения 15", "Ед. изм"=0, "Список"="", "Адрес"=1816, "Описание"="Может использоваться для общих целей. ВНИМАНИЕ! Данная переменная не записывается в энергонезависимую память.", "Мин"=-2147483647, "Макс"=2147483647, "Сервис"=FALSE, "Только чтение"=FALSE, "Разработка"=FALSE, "К-во бит"=32, "Шаг"=0, "Обработка"=FALSE, "Макрос"=""}, {"Имя"="dd32", "Группа"="dd", "Наименование"="Задержка синхронизации", "Ед. изм"=14, "Список"="", "Адрес"=1066, "Описание"="Время между приемом команды упарвления и команды синхронизации. Параметр действителен только для приоводов с интерфейсом упарвления EtherCAT и при активизации управления от СЧПУ.", "Мин"=0, "Макс"=0, "Сервис"=FALSE, "Только чтение"=TRUE, "Разработка"=FALSE, "К-во бит"=32, "Шаг"=0, "Обработка"=FALSE, "Макрос"=""}, {"Имя"="cp11", "Группа"="cp", "Наименование"="Коэффициент ФНЧ входного сигнала", "Ед. изм"=0, "Список"="", "Адрес"=2081, "Описание"="Коэффициент ФНЧ входного сигнала контура тока.", "Мин"=0, "Макс"=1, "Сервис"=TRUE, "Только чтение"=FALSE, "Разработка"=FALSE, "К-во бит"=32, "Шаг"=12, "Обработка"=FALSE, "Макрос"=""}, {"Имя"="cp12", "Группа"="cp", "Наименование"="Коэффициент ФНЧ сигнала ОС", "Ед. изм"=0, "Список"="", "Адрес"=2082, "Описание"="Коэффициент ФНЧ сигнала обратной связи контура тока.", "Мин"=0, "Макс"=1, "Сервис"=TRUE, "Только чтение"=FALSE, "Разработка"=FALSE, "К-во бит"=32, "Шаг"=12, "Обработка"=FALSE, "Макрос"=""}, {"Имя"="st11", "Группа"="st", "Наименование"="Разрешение на полюс двигателя", "Ед. изм"=1, "Список"="", "Адрес"=2083, "Описание"="Формуля для расчета:", "Мин"=1000, "Макс"=2098176, "Сервис"=FALSE, "Только чтение"=FALSE, "Разработка"=FALSE, "К-во бит"=32, "Шаг"=0, "Обработка"=FALSE, "Макрос"=""}, {"Имя"="st12", "Группа"="st", "Наименование"="Коэффициент деления энкодера", "Ед. изм"=0, "Список"="", "Адрес"=2084, "Описание"="Уменьшает разрешение датчика позиции (энкодера) в 2 или 4 раза. Если st12=1, то разрешение энкодера не уменьшается и соответствует физическому разрешению, выдаваемому самим датчиком.", "Мин"=1, "Макс"=4, "Сервис"=FALSE, "Только чтение"=FALSE, "Разработка"=FALSE, "К-во бит"=16, "Шаг"=0, "Обработка"=FALSE, "Макрос"=""}, {"Имя"="st13", "Группа"="st", "Наименование"="Инвертированные сигналы UVW", "Ед. изм"=0, "Список"="0:Нет\n21930:Да\n\r\n", "Адрес"=2085, "Описание"="UVW треки должны следовать в следующем порядке: 2, 3, 1, 5, 4, 6. Для таких датчиков st13=Нет. В некоторых датчиках сигналы идут с инверсией, в этом случае последовательность: 2, 6, 4, 5, 1, 3. Для таких датчиков st13=Да.", "Мин"=-2147483647, "Макс"=2147483647, "Сервис"=FALSE, "Только чтение"=FALSE, "Разработка"=FALSE, "К-во бит"=32, "Шаг"=0, "Обработка"=FALSE, "Макрос"=""}, {"Имя"="dd33", "Группа"="dd", "Наименование"="Кол-во импульсов на сектор UVW сигнала", "Ед. изм"=6, "Список"="", "Адрес"=1067, "Описание"="Кол-во импульсов датчика позиции, приходящееся на текущий сектор UVW сигнала.", "Мин"=-2147483647, "Макс"=2147483647, "Сервис"=FALSE, "Только чтение"=TRUE, "Разработка"=FALSE, "К-во бит"=32, "Шаг"=0, "Обработка"=FALSE, "Макрос"=""}, {"Имя"="dd34", "Группа"="dd", "Наименование"="Ток в роторной системе координат", "Ед. изм"=1, "Список"="", "Адрес"=1068, "Описание"="Ток, пересчитанный в роторную систему координат. Данный сигнал является обратной связью на задание ddd2", "Мин"=-2147483647, "Макс"=2147483647, "Сервис"=TRUE, "Только чтение"=TRUE, "Разработка"=FALSE, "К-во бит"=32, "Шаг"=12, "Обработка"=FALSE, "Макрос"=""}, {"Имя"="st14", "Группа"="st", "Наименование"="Автоматический поиск фазы", "Ед. изм"=0, "Список"="0:Фаза не найдена\n170:Запрос поиска фазы\n171:Ожидание завершения поиска фазы\n172:Ожидаем вращения в +\n173:Ожидаем вращения в -\n174:Ошибка поиска\n175:Поиск выполнен успешно\n\r\n", "Адрес"=2086, "Описание"="Параметр используется для отображения текущего состояния поиска фазы в автоматическом режиме. Поиск фазы позволяет настроить сервоусилитель на конкретный экземпляр двигателя.", "Мин"=0, "Макс"=175, "Сервис"=FALSE, "Только чтение"=TRUE, "Разработка"=FALSE, "К-во бит"=16, "Шаг"=0, "Обработка"=FALSE, "Макрос"=""}] {"Ед. изм" items=["", "дискрет", "об/(сек^2)", "сек", "об/мин", "А", "имп.", "град.", "В", "мксек", "Банк", "мсек", "кГц", "А2сек", "nсек"]; "Адрес" format="%04x"}
  in  "Имена парам":cluster{string[]}[](array[cluster])
  in  "Параметр":u16(ring) items=["dd1", "dd10", "dd11", "dd12", "dd13", "dd14", "dd15", "dd16", "dd17", "dd18", "dd19", "dd2", "dd20", "dd21", "dd22", "dd23", "dd24", "dd25", "dd26", "dd27", "dd28", "dd29", "dd3", "dd30", "dd31", "dd32", "dd33", "dd34", "dd4", "dd5", "dd6", "dd7", "dd8", "dd9"]
  in  "Группа":u16(ring) items=["cp", "ct", "dd", "ep", "io", "ip", "pd", "pp", "ss", "st", "tp", "up", "vp"]
  in  "Группы":string[](array[string])
  out "Ответ полный":u8[](array[numeric]) format="%02x"
  out "Ответ расшифрованный":u8[](array[numeric]) format="%02x"
  out "error out":errorcluster
  out "Запрос симв.":string
  in  "VISA name":refnum<visa-resource-name>="COM6"
  in  "Пуск":bool
  in  "Выход":bool
  out "Запрос зашифрованный":u8[](array[numeric])=[1, 5, 0, 30, 0, 0, 0, 0, 3] format="%02x"
  out "return count":u32
  out "Ответ симв.":string
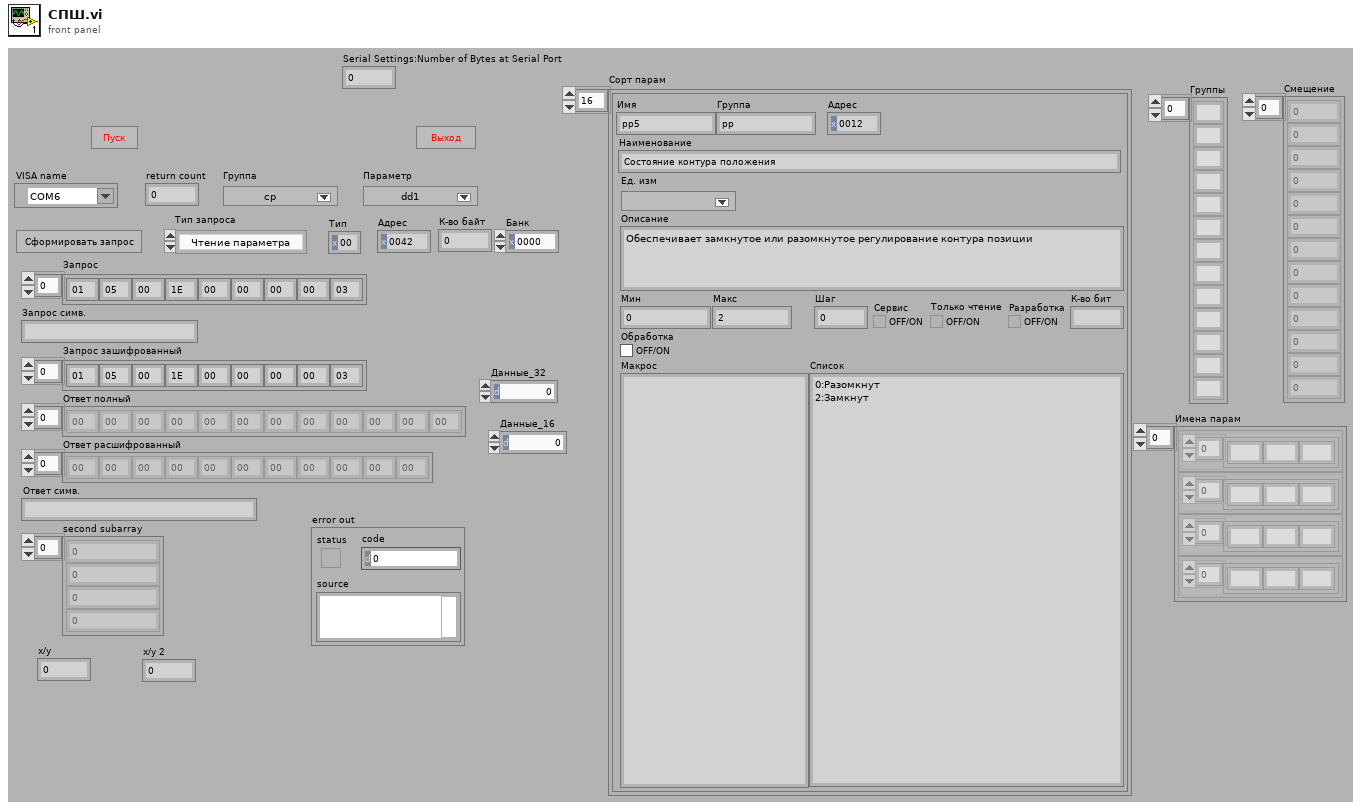
[diagram p1: front panel]
types:
  T1 = enum16{"Чтение параметра ", "Запись параметра", "Запуск программы ПЛК"}
  T2 = cluster{"Имя":string, "Группа":string, "Наименование":string, "Ед. изм":u16, "Список":string, "Адрес":u32, "Описание":string, "Мин":i32, "Макс":i32, "Сервис":bool, "Только чтение":bool, "Разработка":bool, "К-во бит":u16, "Шаг":u32, "Обработка":bool, "Макрос":string}[]
  T3 = cluster{"Имя":string, "Группа":string, "Наименование":string, "Ед. изм":u16, "Список":string, "Адрес":u32, "Описание":string, "Мин":i32, "Макс":i32, "Сервис":bool, "Только чтение":bool, "Разработка":bool, "К-во бит":u16, "Шаг":u32, "Обработка":bool, "Макрос":string}
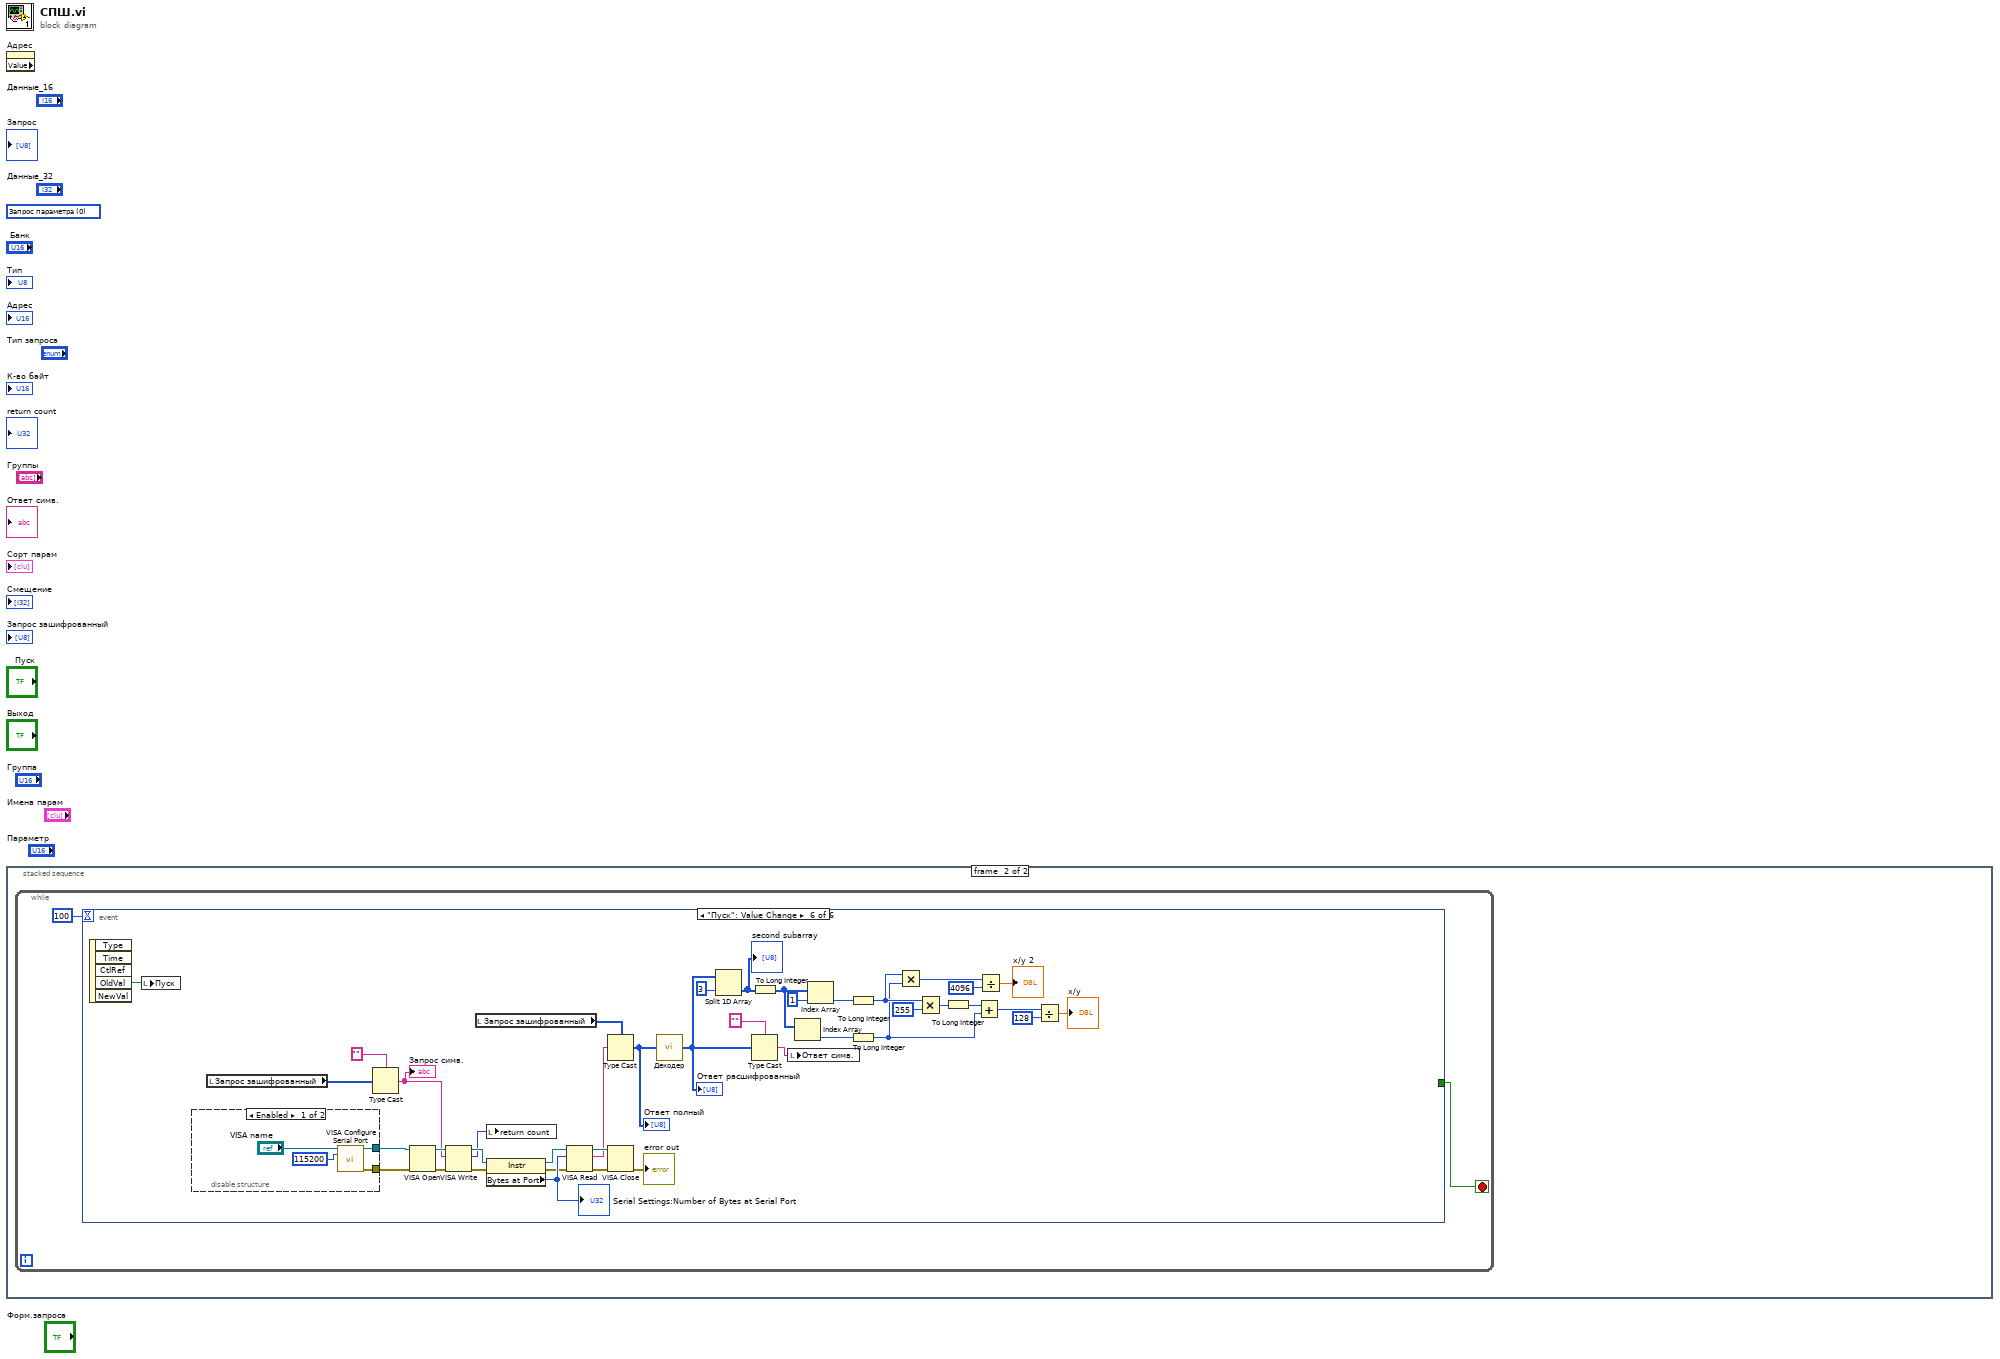
[diagram p0: block diagram]
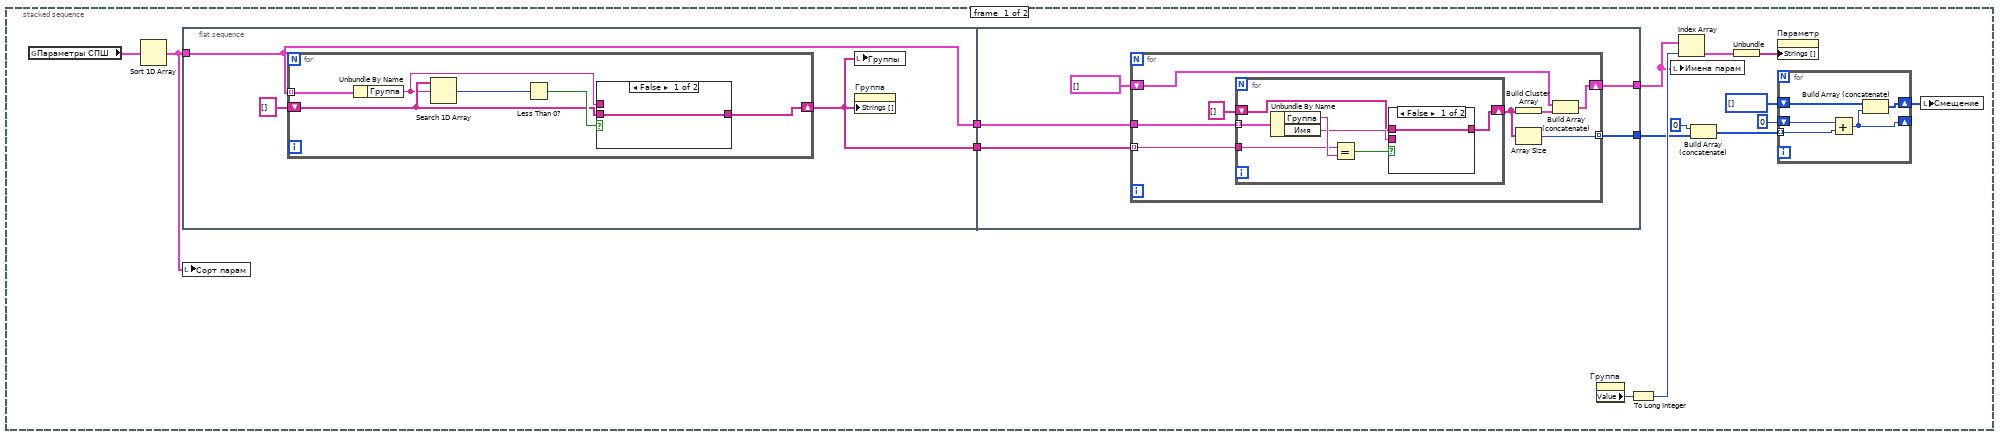
[diagram p2: hidden frame]
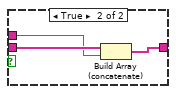
[diagram p3: hidden frame]
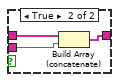
[diagram p4: hidden frame]
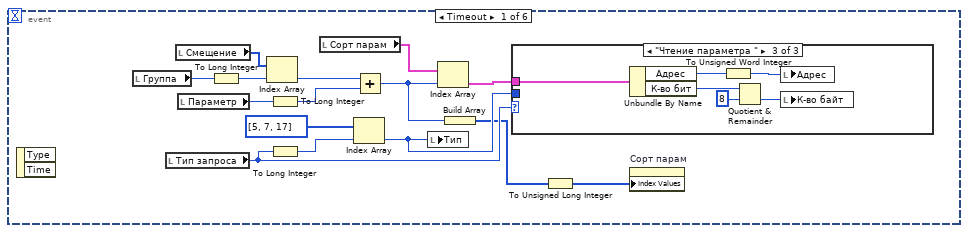
[diagram p5: hidden frame]
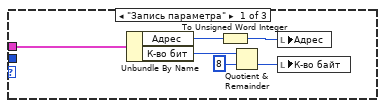
[diagram p6: hidden frame]
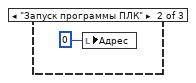
[diagram p7: hidden frame]
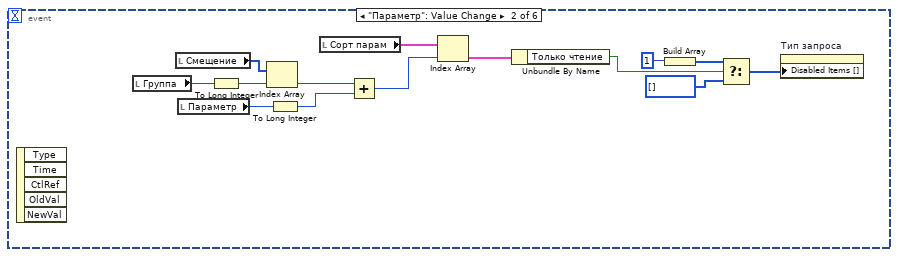
[diagram p8: hidden frame]
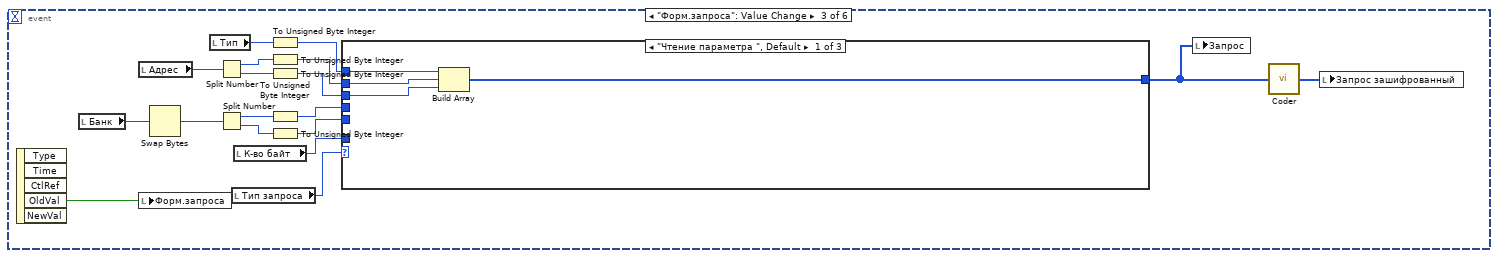
[diagram p9: hidden frame]
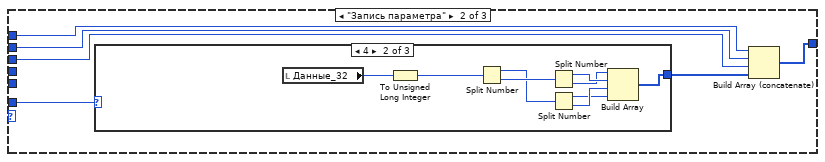
[diagram p10: hidden frame]
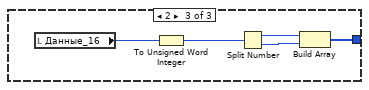
[diagram p12: hidden frame]
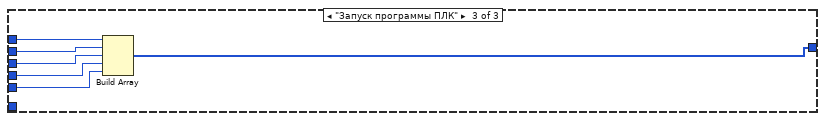
[diagram p13: hidden frame]
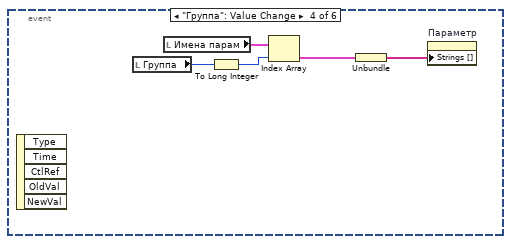
[diagram p14: hidden frame]
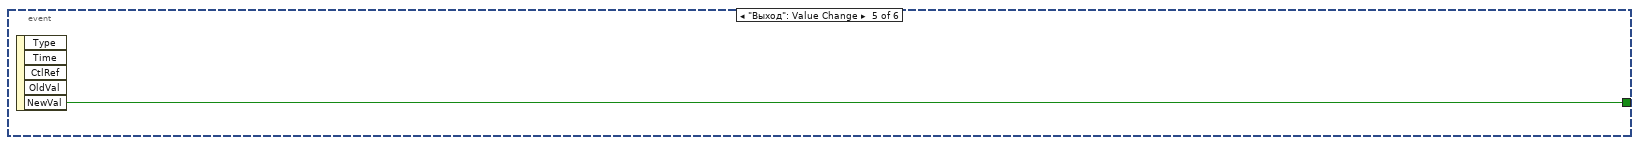
[diagram p15: hidden frame]
diagram:
  (unwired) u16 0 items=["Запрос параметра ", "Чтение параметра", "Запись параметра", "Запуск программы ПЛК"] ("Тип запроса")
  n1 = property on="Адрес" class="DigNum (strict)" props=["Value"]() -> ()  [unwired: 2 in, 3 out]
  n2 = stacked-sequence {
    frame #0 {
      n3 = global read "Параметры СПШ.vi" "Параметры СПШ"() -> (w11:T2)
      n4 = Sort 1D Array(array=w11) -> (sorted array=w6:T2)
      n5 = flat-sequence {
        tunnel: w6 -> [w17]
        tunnel: [w16] -> w5
        tunnel: [w17] -> w4
        tunnel: w5 -> [w32]
        tunnel: w4 -> [w31]
        tunnel: [w30] -> w3
        tunnel: [w29] -> w2
        frame #0 {
          n6 = for {
            tunnel: w17 -> [w24] mode=indexing
            shift-right: [w20] -> w16
            shift-left: string[] [] -> [w21]
            n7 = Unbundle By Name(w24) -> ("Группа"=w19:string)
            n8 = Search 1D Array(1D array=w21, element=w19) -> (index of element=w23:i32)  [unwired: 1 in]
            n9 = Less Than 0?(x=w23) -> (x < 0?=w22:bool)
            n10 = case shown="False" w22 {
              tunnel: w21 -> [w25 w28]
              tunnel: [w25 w27] -> w20
              tunnel: w19 -> [_ w26]
              frame False {
              }
              frame True {
                n11 = Build Array (concatenate)(w28, w26) -> (w27:string[])
              }
            }
          }
          n12 = local write "Группы"(w16) -> ()
          n13 = property on="Группа" class="Ring (strict)"("Strings []"=w16) -> ()  [unwired: 2 in, 2 out]
        }
        frame #1 {
          n14 = for {
            tunnel: w32 -> [w40] mode=indexing
            tunnel: w31 -> [w41]
            shift-right: [w36] -> w29
            shift-left: cluster{string[]}[] [] ("array of clusters") -> [w37]
            tunnel: [w34] -> w30 mode=indexing
            n15 = for {
              tunnel: w41 -> [w48] mode=indexing
              tunnel: w40 -> [w46]
              shift-right: [w42] -> w35
              shift-left: string[] [] -> [w43]
              n16 = Unbundle By Name(w48) -> ("Группа"=w47:string, "Имя"=w44:string)
              n17 = Equal?(x=w46, y=w47) -> (x = y?=w45:bool)
              n18 = case shown="False" w45 {
                tunnel: w44 -> [_ w52]
                tunnel: w43 -> [w49 w51]
                tunnel: [w49 w50] -> w42
                frame False {
                }
                frame True {
                  n19 = Build Array (concatenate)(w51, w52) -> (w50:string[])
                }
              }
            }
            n20 = Build Cluster Array(w35) -> (w38:cluster{string[]}[])
            n21 = Array Size(array=w35) -> (size(s)=w34:i32)
            n22 = Build Array (concatenate)(w37, w38) -> (w36:cluster{string[]}[])
          }
        }
      }
      n23 = local write "Сорт парам"(w6) -> ()
      n24 = property on="Группа" class="Ring (strict)"() -> ("Value"=w15:u16)  [unwired: 2 in, 2 out]
      n25 = To Long Integer(number=w15) -> (32bit integer=w12:i32)
      n26 = local write "Имена парам"(w2) -> ()
      n27 = Index Array(array=w2, index=w12) -> (element=w14:cluster{string[]})
      n28 = Build Array (concatenate)(0, w3) -> (w9:i32[])
      n29 = Unbundle(w14) -> (w13:string[])
      n30 = property on="Параметр" class="Ring (strict)"("Strings []"=w13) -> ()  [unwired: 2 in, 2 out]
      n31 = for {
        tunnel: w9 -> [w54] mode=indexing
        shift-right: [w56] -> w7
        shift-left: i32[] [] -> [w57]
        shift-right: [w55] -> _
        shift-left: 0 -> [w53]
        n32 = Add(x=w53, y=w54) -> (x+y=w55:i32)
        n33 = Build Array (concatenate)(w57, w55) -> (w56:i32[])
      }
      n34 = local write "Смещение"(w7) -> ()
    }
    frame #1 {
      n35 = while {
        stop <- w59 stop-if-true
        n36 = event shown="[5] \"Пуск\": Value Change" {
          selector: _ -> [_ _ _ _ _ _]
          dyn-events: _ -> [_ _ _ _ _ _]
          timeout: 100 -> [_ _ _ _ _ _]
          tunnel: [_ _ _ _ w155 _] -> w59
          event Timeout {
            n37 = event-data() -> ()  [unwired: 1 in, 2 out]
            n38 = local read "Группа"() -> (w68:u16)
            n39 = local read "Тип запроса"() -> (w72:T1)
            n40 = local read "Смещение"() -> (w65:i32[])
            n41 = local read "Параметр"() -> (w69:u16)
            n42 = To Long Integer(number=w68) -> (32bit integer=w66:i32)
            n43 = Index Array(array=w65, index=w66) -> (element=w67:i32)
            n44 = To Long Integer(number=w69) -> (32bit integer=w70:i32)
            n45 = To Long Integer(number=w72) -> (32bit integer=w73:i32)
            n46 = local read "Сорт парам"() -> (w64:T2)
            n47 = Index Array(array=u8[] [5, 7, 17], index=w73) -> (element=w71:u8)
            n48 = Add(x=w67, y=w70) -> (x+y=w61:i32)
            n49 = local write "Тип"(w71) -> ()
            n50 = Index Array(array=w64, index=w61) -> (element=w60:T3)
            n51 = Build Array(w61) -> (w62:i32[])
            n52 = case shown="\"Чтение параметра \"" w72 {
              tunnel: w71 -> [_ _ _]
              tunnel: w60 -> [w75 _ w83]
              frame "Запись параметра" {
                n53 = Unbundle By Name(w75) -> ("Адрес"=w80:u32, "К-во бит"=w79:u16)
                n54 = To Unsigned Word Integer(number=w80) -> (unsigned 16bit integer=w76:u16)
                n55 = Quotient & Remainder(x=w79, y=u16 8) -> (floor(x/y)=w77:u16)  [unwired: 1 out]
                n56 = local write "Адрес"(w76) -> ()
                n57 = local write "К-во байт"(w77) -> ()
              }
              frame "Запуск программы ПЛК" {
                n58 = local write "Адрес"(u32 0 ("Адрес")) -> ()
              }
              frame "Чтение параметра " {
                n59 = Unbundle By Name(w83) -> ("Адрес"=w87:u32, "К-во бит"=w86:u16)
                n60 = To Unsigned Word Integer(number=w87) -> (unsigned 16bit integer=w82:u16)
                n61 = Quotient & Remainder(x=w86, y=u16 8) -> (floor(x/y)=w84:u16)  [unwired: 1 out]
                n62 = local write "Адрес"(w82) -> ()
                n63 = local write "К-во байт"(w84) -> ()
              }
            }
            n64 = To Unsigned Long Integer(number=w62) -> (unsigned 32bit integer=w63:u32[])
            n65 = property on="Сорт парам" class="Arr (strict)"("Index Values"=w63) -> ()  [unwired: 2 in, 2 out]
          }
          event "Параметр": Value Change {
            n66 = event-data() -> ()  [unwired: 1 in, 5 out]
            n67 = local read "Группа"() -> (w100:u16)
            n68 = local read "Смещение"() -> (w101:i32[])
            n69 = local read "Параметр"() -> (w97:u16)
            n70 = To Long Integer(number=w100) -> (32bit integer=w99:i32)
            n71 = Index Array(array=w101, index=w99) -> (element=w98:i32)
            n72 = To Long Integer(number=w97) -> (32bit integer=w95:i32)
            n73 = local read "Сорт парам"() -> (w94:T2)
            n74 = Add(x=w98, y=w95) -> (x+y=w96:i32)
            n75 = Index Array(array=w94, index=w96) -> (element=w93:T3)
            n76 = Unbundle By Name(w93) -> ("Только чтение"=w92:bool)
            n77 = Build Array(1) -> (w90:i32[])
            n78 = Select(t=w90, s=w92, f=i32[] []) -> (s? t:f=w88:i32[])
            n79 = property on="Тип запроса" class="Enum (strict)"("Disabled Items []"=w88) -> ()  [unwired: 2 in, 2 out]
          }
          event "Форм.запроса": Value Change {
            n80 = event-data() -> ("OldVal"=w119:bool)  [unwired: 1 in, 4 out]
            n81 = local read "Банк"() -> (w105:u16)
            n82 = local read "Адрес"() -> (w106:u16)
            n83 = local write "Форм.запроса"(w119) -> ()
            n84 = Swap Bytes(anything=w105) -> (byte swapped=w104:u16)
            n85 = local read "Тип"() -> (w116:u8)
            n86 = Split Number(x=w106) -> (hi(x)=w113:u8, lo(x)=w114:u8)
            n87 = Split Number(x=w104) -> (hi(x)=w110:u8, lo(x)=w109:u8)
            n88 = local read "Тип запроса"() -> (w102:T1)
            n89 = local read "К-во байт"() -> (w103:u16)
            n90 = To Unsigned Byte Integer(number=w116) -> (unsigned 8bit integer=w115:u8)
            n91 = To Unsigned Byte Integer(number=w113) -> (unsigned 8bit integer=w112:u8)
            n92 = To Unsigned Byte Integer(number=w114) -> (unsigned 8bit integer=w111:u8)
            n93 = To Unsigned Byte Integer(number=w110) -> (unsigned 8bit integer=w108:u8)
            n94 = To Unsigned Byte Integer(number=w109) -> (unsigned 8bit integer=w107:u8)
            n95 = case shown="\"Чтение параметра \", Default" w102 {
              tunnel: [w123 w126 w144] -> w117
              tunnel: w115 -> [w122 w129 w149]
              tunnel: w112 -> [w120 w128 w148]
              tunnel: w111 -> [w121 w127 w147]
              tunnel: w108 -> [_ _ w146]
              tunnel: w107 -> [_ _ w145]
              tunnel: w103 -> [_ w125 _]
              frame "Чтение параметра ", Default {
                n96 = Build Array(w122, w120, w121) -> (w123:u8[])
              }
              frame "Запись параметра" {
                n97 = case shown="4" w125 {
                  tunnel: [_ w136 w140] -> w124
                  frame 0, Default {
                  }
                  frame 4 {
                    n98 = local read "Данные_32"() -> (w138:i32)
                    n99 = To Unsigned Long Integer(number=w138) -> (unsigned 32bit integer=w137:u32)
                    n100 = Split Number(x=w137) -> (hi(x)=w134:u16, lo(x)=w135:u16)
                    n101 = Split Number(x=w135) -> (hi(x)=w131:u8, lo(x)=w130:u8)
                    n102 = Split Number(x=w134) -> (hi(x)=w132:u8, lo(x)=w133:u8)
                    n103 = Build Array(w130, w131, w133, w132) -> (w136:u8[])
                  }
                  frame 2 {
                    n104 = local read "Данные_16"() -> (w143:i16)
                    n105 = To Unsigned Word Integer(number=w143) -> (unsigned 16bit integer=w139:u16)
                    n106 = Split Number(x=w139) -> (hi(x)=w142:u8, lo(x)=w141:u8)
                    n107 = Build Array(w142, w141) -> (w140:u8[])
                  }
                }
                n108 = Build Array (concatenate)(w129, w128, w127, w124) -> (w126:u8[])
              }
              frame "Запуск программы ПЛК" {
                n109 = Build Array(w149, w148, w147, w146, w145) -> (w144:u8[])
              }
            }
            n110 = local write "Запрос"(w117) -> ()
            n111 = call "Coder.vi"("Запрос Вх"=w117) -> ("Запрос Вых"=w118:u8[])
            n112 = local write "Запрос зашифрованный"(w118) -> ()
          }
          event "Группа": Value Change {
            n113 = event-data() -> ()  [unwired: 1 in, 5 out]
            n114 = local read "Группа"() -> (w150:u16)
            n115 = local read "Имена парам"() -> (w152:cluster{string[]}[])
            n116 = To Long Integer(number=w150) -> (32bit integer=w151:i32)
            n117 = Index Array(array=w152, index=w151) -> (element=w154:cluster{string[]})
            n118 = Unbundle(w154) -> (w153:string[])
            n119 = property on="Параметр" class="Ring (strict)"("Strings []"=w153) -> ()  [unwired: 2 in, 2 out]
          }
          event "Выход": Value Change {
            n120 = event-data() -> ("NewVal"=w155:bool)  [unwired: 1 in, 4 out]
          }
          event "Пуск": Value Change {
            n121 = event-data() -> ("OldVal"=w175:bool)  [unwired: 1 in, 4 out]
            n122 = local write "Пуск"(w175) -> ()
            n123 = disable-structure shown="Enabled" {
              disable-tunnel: [w199 _] -> w176
              disable-tunnel: [w196 _] -> w177
              frame Enabled {
                n124 = call-poly "VISA Configure Serial Port"("VISA resource name"="VISA name", "baud rate (9600)"=u32 115200) -> ("VISA resource name out"=w199:refnum<visa-resource-name>, "error out"=w196:errorcluster)  [unwired: 12 in]
              }
              frame Disabled {
              }
            }
            n125 = local read "Запрос зашифрованный"() -> (w181:u8[])
            n126 = Type Cast(type="" ("write buffer"), x=w181) -> (*(type *) &x=w179:string)
            "Запрос симв." <- w179
            n127 = VISA Open(error in (no error)=w177, VISA resource name=w176) -> (VISA resource name=w183:refnum<visa-resource-name>, error out=w184:errorcluster)  [unwired: 3 in]
            n128 = VISA Write(VISA resource name=w183, write buffer=w179, error in (no error)=w184) -> (VISA resource name out=w185:refnum<visa-resource-name>, return count=w182:u32, error out=w187:errorcluster)
            n129 = local read "Запрос зашифрованный"() -> (w191:u8[])
            n130 = local write "return count"(w182) -> ()
            n131 = property class="Instr"(reference=w185, error in=w187) -> (reference out=w186:refnum<visa-resource-name>, error out=w188:errorcluster, "Bytes at Port"=w189:u32)
            "Serial Settings:Number of Bytes at Serial Port" <- w189
            n132 = VISA Read(VISA resource name=w186, byte count=w189, error in (no error)=w188) -> (VISA resource name out=w194:refnum<visa-resource-name>, read buffer=w190:string, error out=w195:errorcluster)  [unwired: 1 out]
            n133 = Type Cast(type=w191, x=w190) -> (*(type *) &x=w164:u8[])
            "Ответ полный" <- w164
            n134 = VISA Close(VISA resource name=w194, error in (no error)=w195) -> (error out=→"error out":errorcluster)
            n135 = call "Декодер.vi"("Ответ Вх"=w164) -> ("Ответ Вых"=w163:u8[])
            "Ответ расшифрованный" <- w163
            n136 = Split 1D Array(array=w163, index=3) -> (second subarray=w173:u8[])  [unwired: 1 out]
            "second subarray" <- w173
            n137 = To Long Integer(number=w173) -> (32bit integer=w162:i32[])
            n138 = Type Cast(type="" ("write buffer"), x=w163) -> (*(type *) &x=w193:string)
            n139 = local write "Ответ симв."(w193) -> ()
            n140 = Index Array(array=w162) -> (element=w160:i32)  [unwired: 1 in]
            n141 = Index Array(array=w162, index=1) -> (element=w172:i32)
            n142 = To Long Integer(number=w172) -> (32bit integer=w161:i32)
            n143 = To Long Integer(number=w160) -> (32bit integer=w159:i32)
            n144 = Multiply(x=w161, y=w159) -> (x*y=w158:i32)
            n145 = Multiply(x=w161, y=255) -> (x*y=w170:i32)
            n146 = To Long Integer(number=w170) -> (32bit integer=w165:i32)
            n147 = Add(x=w165, y=w159) -> (x+y=w169:i32)
            n148 = Divide(x=w158, y=4096) -> (x/y=→"x/y 2":dbl)
            n149 = Divide(x=w169, y=128) -> (x/y=→"x/y":dbl)
          }
        }
      }
    }
  }
